vi "commander11.vi"() -> ()   [LabVIEW 2015]
uses:
  <vilib>/National Instruments/NI Dynamixel API/Dynamixel Pro Driver/Controls/Write Select Pro.ctl
  <vilib>/National Instruments/NI Dynamixel API/Dynamixel Pro Driver/Controls/Baudrate Selector.ctl
  G_LCM.vi
  G_ALL.vi
  G_SEN.vi
  <vilib>/National Instruments/NI Dynamixel API/Dynamixel Pro Driver/Write/Write Dynamixel Pro.vi
  <vilib>/National Instruments/NI Dynamixel API/Dynamixel Pro Driver/Helper VIs/Torque Disable.vi
  <vilib>/National Instruments/NI Dynamixel API/Dynamixel Pro Driver/Helper VIs/Torque Enable.vi
  <vilib>/National Instruments/NI Dynamixel API/Dynamixel Pro Driver/Dynamixel Pro Driver.lvlib
panel:
  in  "an":dbl=0.1 format="%#_13g"
  out "Mobileye":bool=TRUE
  in  "Laser lane":bool
  in  "safe  dist":dbl=0.7 format="%#_13g"
  in  "Path Num":i32=1 min=1 max=5 step=1
  out "CIPV_SPEED":dbl=25.0
  out "CIPV_dist":dbl=25.0
  in  "mission":i32
  out "size(s)":i32=1381
  in  "shift torque gain":i32
  out "robotis":refnum<visa-resource-name>
  in  "y 2":dbl=1.0
  in  "y":dbl=0.5 format="%#_13g"
  in  "dist_error_gain":dbl=0.5 format="%#_13g"
  in  "Global y shift":dbl min=-5.0 max=5.0 step=0.1
  in  "d":dbl=-3.5 format="%#_13g"
  in  "reset path":bool
  out "count":i32=100
  out "signal":picture[](array[picture])=[bytes[7530], bytes[7530], bytes[7530], bytes[7530]]
  out "sign":picture[](array[picture])=[bytes[7530], bytes[7530], bytes[7530], bytes[7530]]
  out "trafic signal ref":picture[](array[picture])=[bytes[7530], bytes[7530], bytes[7530], bytes[7530], bytes[7530], bytes[7530]]
  out "sign ref":picture[](array[picture])=[bytes[7530], bytes[7530], bytes[7530], bytes[7530], bytes[7530], bytes[7530], bytes[7530], bytes[7530], bytes[7530], bytes[7530], bytes[7530], bytes[7530], bytes[7530]]
  in  "TTL":bool=TRUE
  in  "lane keep":bool
  in  "replay":bool
  in  "Global x shift":dbl min=-5.0 max=5.0 step=1.0
  out "display":u32=33 format="%02.0f"
  out "control":u32=10 format="%02.0f"
  in  "Vision Lane":bool=TRUE
  in  "save lcm":bool
  out "LCM Recv Data":string
  out "GPS DATA 2":T1={"type"="None", "x_lcc"=0.0, "y_lcc"=0.0, "latdev"=0.0, "londev"=0.0, "sats"=0, "gps_l1_ranges"=0, "gps_l1_mask_ranges"=0, "gps_l2_mask_ranges"=0, "Heading"=0.0, "lon"=0.0, "lat"=0.0, "time"="09:00:00.0", "hgps"=0.0, "lag"=0.0, "MAP"=""} {"lag" format="%#_5g"; "hgps" format="%#_5g"; "lat" format="%#_11g"; "lon" format="%#_11g"; "Heading" format="%#_5g"; "latdev" format="%#_4g"; "londev" format="%#_4g"}
  in  "Obs":bool=TRUE
  in  "Log":bool
  out "path":u32=10 format="%02.0f"
  out "sensor":u32=27 format="%02.0f"
  out "Speed limit":dbl=10.0
  out "collision":bool
  in  "Load Path":bool
  in  "Max. Vel.":dbl=10.0 min=-5.0 max=120.0 step=5.0
  out "col":i16(graph)
  out "stop":bool
  in  "Reverse":bool
  in  "STOP":bool
  out "Waveform Chart 4":cluster{"auto":i16, "run":i16}(graph)={"auto"=1, "run"=0}
  out "Waveform Chart 3":cluster{"Steer_input":dbl, dbl, "handle":dbl}(graph)={"Steer_input"=0.0, -0.0, "handle"=nan}
  out "Waveform Chart 2":T2(graph)={"VS_des"=0.0, "VS_can"=0.0, "VS_des"=10.0}
  out "Heading":cluster{"Heading":dbl, "hgps":dbl}(graph)
  out "XY Graph 2":cluster{"Y":dbl[], "Y":dbl[]}[](graph)
  out "Gauge":cluster{dbl, dbl, dbl}(knob)={0.0, 0.0, 10.0} scale=-20.0..140.0
  out "Meter":cluster{dbl, dbl, dbl}(knob)={0.0, -0.0, nan} scale=-550.0..550.0
  out "XY Graph":cluster{"Y":dbl[], "Y":dbl[]}[](graph)=[{"Y"=[], "Y"=[]}, {"Y"=[-0.0, -0.0, -0.0, -0.0, -0.0, -0.0, -0.0, -0.0, -0.0, -0.0, -0.0, -0.0, -0.0, -0.0, -0.0, -0.0, -0.0, -0.0, -0.0, -0.0, -0.0, -0.0, -0.0, -0.0, -0.0, -0.0, -0.0, -0.0, -0.0, -0.0, -0.0], "Y"=[-4.0, -3.9, -3.8, -3.7, -3.6, -3.5, -3.4, -3.3, -3.2, -3.1, -3.0, -2.9, -2.8, -2.7, -2.5999999999999996, -2.5, -2.4, -2.3, -2.2, -2.0999999999999996, -2.0, -1.9, -1.7999999999999998, -1.6999999999999997, -1.5999999999999996, -1.5, -1.4, -1.2999999999999998, -1.1999999999999997, -1.0999999999999996, -1.0]}, {"Y"=[0.0], "Y"=[0.0]}, {"Y"=[], "Y"=[]}, {"Y"=[-0.925, -0.925, -0.925, -0.6775, -0.6775, -0.925, -0.925, -0.925, -0.925, -0.6775, -0.6775, -0.925, -0.925, -0.925, 0.9025, 0.9025, 0.9025, 0.6775, 0.6775, 0.9025, 0.9025, 0.9025, 0.9025, 0.6775, 0.6775, 0.9025, 0.9025, 0.9025, -0.925], "Y"=[-0.75, -0.224, 0.224, 0.224, -0.224, -0.224, 0.224, 2.415, 2.885, 2.885, 2.415, 2.415, 2.885, 3.5, 3.5, 2.885, 2.415, 2.415, 2.885, 2.885, 2.415, 0.224, -0.224, -0.224, 0.224, 0.224, -0.224, -0.75, -0.75]}, {"Y"=[-0.11693930899008871, -0.11530935243371389, -0.11366872898963808, -0.11201743865786128, -0.11035548143838347, -0.10868285733120467, -0.10699956633632488, -0.10530560845374409, -0.1036009836834623, -0.10188569202547951, -0.10015973347979573, -0.09842310804641094, -0.09667581572532517, -0.09491785651653842, -0.09314923042005063, -0.09136993743586189, -0.08957997756397212, -0.08777935080438137, -0.08596805715708963, -0.08414609662209688, -0.08231346919940313, -0.0804701748890084, -0.07861621369091265, -0.07675158560511593, -0.07487629063161819, -0.07299032877041947, -0.07109370002151975, -0.06918640438491905, -0.06726844186061733, -0.06533981244861461, -0.06340051614891093, -0.061450552961506213, -0.05948992288640052, -0.05751862592359382, -0.055536662073086135, -0.05354403133487746, -0.05154073370896778, -0.0495267691953571, -0.04750213779404542, -0.045466839505032754, -0.04342087432831909, -0.04136424226390442, -0.03929694331178877, -0.03721897747197212, -0.035130344744454464, -0.033031045129235825, -0.03092107862631617, -0.028800445235695537, -0.02666914495737389, -0.024527177791351266, -0.02237454373762765, -0.02021124279620301, -0.018037274967077403, -0.015852640250250776, -0.013657338645723171, -0.011451370153494574, -0.009234734773564957, -0.007007432505934365, -0.004769463350602757, -0.002520827307570167, -0.0002615243768365888, 0.0020084454415980058, 0.004289082147733582, 0.0065803857415701675, 0.008882356223107735, 0.011194993592346297, 0.013518297849285876, 0.01585226899392643, 0.018196907026268, 0.020552211946310545, 0.02291818375405409, 0.025294822449498655, 0.02768212803264418, 0.03008010050349072, 0.03248873986203825, 0.03490804610828678, 0.037338019242236314, 0.03977865926388684, 0.04222996617323836, 0.044691939970290875, 0.04716458065504438, 0.04964788822749888, 0.05214186268765442, 0.05464650403551091, 0.057161812271068396, 0.05968778739432688, 0.06222442940528636, 0.06477173830394688, 0.06732971409030836, 0.06989835676437083, 0.07247766632613428, 0.07506764277559874, 0.07766828611276426, 0.08027959633763071, 0.08290157345019813, 0.08553421745046658, 0.08817752833843606, 0.09083150611410651, 0.09349615077747794, 0.09617146232855037, 0.0988574407673238], "Y"=[-4.0, -3.9, -3.8, -3.7, -3.6, -3.5, -3.4, -3.3, -3.2, -3.1, -3.0, -2.9, -2.8, -2.7, -2.5999999999999996, -2.5, -2.4, -2.3, -2.2, -2.0999999999999996, -2.0, -1.9, -1.7999999999999998, -1.6999999999999997, -1.5999999999999996, -1.5, -1.4, -1.2999999999999998, -1.1999999999999997, -1.0999999999999996, -1.0, -0.8999999999999999, -0.7999999999999998, -0.6999999999999997, -0.5999999999999996, -0.5, -0.3999999999999999, -0.2999999999999998, -0.19999999999999973, -0.09999999999999964, 0.0, 0.10000000000000053, 0.20000000000000018, 0.2999999999999998, 0.40000000000000036, 0.5, 0.6000000000000005, 0.7000000000000002, 0.8000000000000007, 0.9000000000000004, 1.0, 1.1000000000000005, 1.2000000000000002, 1.3000000000000007, 1.4000000000000004, 1.5, 1.6000000000000005, 1.7000000000000002, 1.8000000000000007, 1.9000000000000004, 2.0, 2.1000000000000005, 2.2, 2.3000000000000007, 2.4000000000000004, 2.5, 2.6000000000000005, 2.7, 2.8000000000000007, 2.9000000000000004, 3.0, 3.1000000000000005, 3.2, 3.3000000000000007, 3.4000000000000004, 3.5, 3.6000000000000005, 3.7, 3.8000000000000007, 3.9000000000000004, 4.0, 4.1, 4.200000000000001, 4.300000000000001, 4.4, 4.5, 4.6, 4.700000000000001, 4.800000000000001, 4.9, 5.0, 5.1, 5.200000000000001, 5.300000000000001, 5.4, 5.5, 5.600000000000001, 5.700000000000001, 5.800000000000001, 5.9, 6.0]}, {"Y"=[0.8254985256386238, 0.8528194590155173, 0.8796538166129886, 0.9060015984310377, 0.9318628044696647, 0.9572374347288698, 0.9821254892086528, 1.0065269679090136, 1.0304418708299523, 1.0538701979714689, 1.0768119493335635, 1.099267124916236, 1.1212357247194864, 1.1427177487433147, 1.163713196987721, 1.184222069452705, 1.204244366138267, 1.2237800870444069, 1.2428292321711245, 1.2613918015184205, 1.279467795086294, 1.2970572128747455, 1.314160054883775, 1.3307763211133825, 1.3469060115635676, 1.3625491262343308, 1.3777056651256718, 1.392375628237591, 1.4065590155700878, 1.4202558271231627, 1.4334660628968152, 1.4461897228910459, 1.4584268071058544, 1.4701773155412408, 1.4814412481972052, 1.4922186050737474, 1.5025093861708676, 1.5123135914885657, 1.5216312210268417, 1.5304622747856955, 1.5388067527651272, 1.546664654965137, 1.5540359813857245, 1.56092073202689, 1.5673189068886335, 1.5732305059709548, 1.578655529273854, 1.583593976797331, 1.5880458485413862, 1.592011144506019, 1.5954898646912299, 1.5984820090970187, 1.6009875777233853, 1.60300657057033, 1.6045389876378524, 1.605584828925953, 1.606144094434631, 1.6062167841638872, 1.6058028981137213, 1.6049024362841335, 1.6035153986751234, 1.601641785286691, 1.599281596118837, 1.5964348311715606, 1.5931014904448622, 1.5892815739387416, 1.584975081653199, 1.5801820135882343, 1.5749023697438473, 1.5691361501200385, 1.5628833547168075, 1.5561439835341544, 1.5489180365720792, 1.541205513830582, 1.5330064153096625, 1.5243207410093211, 1.5151484909295576, 1.505489665070372, 1.4953442634317642, 1.4847122860137343, 1.4735937328162825, 1.4619886038394085, 1.4498968990831123, 1.437318618547394, 1.4242537622322538, 1.4107023301376915, 1.396664322263707, 1.3821397386103003, 1.3671285791774717, 1.351630843965221, 1.335646532973548, 1.3191756462024533, 1.302218183651936, 1.284774145321997, 1.2668435312126356, 1.2484263413238526, 1.229522575655647, 1.2101322342080194, 1.19025531698097, 1.1698918239744982, 1.1490417551886045], "Y"=[-4.0, -3.9, -3.8, -3.7, -3.6, -3.5, -3.4, -3.3, -3.2, -3.1, -3.0, -2.9, -2.8, -2.7, -2.5999999999999996, -2.5, -2.4, -2.3, -2.2, -2.0999999999999996, -2.0, -1.9, -1.7999999999999998, -1.6999999999999997, -1.5999999999999996, -1.5, -1.4, -1.2999999999999998, -1.1999999999999997, -1.0999999999999996, -1.0, -0.8999999999999999, -0.7999999999999998, -0.6999999999999997, -0.5999999999999996, -0.5, -0.3999999999999999, -0.2999999999999998, -0.19999999999999973, -0.09999999999999964, 0.0, 0.10000000000000053, 0.20000000000000018, 0.2999999999999998, 0.40000000000000036, 0.5, 0.6000000000000005, 0.7000000000000002, 0.8000000000000007, 0.9000000000000004, 1.0, 1.1000000000000005, 1.2000000000000002, 1.3000000000000007, 1.4000000000000004, 1.5, 1.6000000000000005, 1.7000000000000002, 1.8000000000000007, 1.9000000000000004, 2.0, 2.1000000000000005, 2.2, 2.3000000000000007, 2.4000000000000004, 2.5, 2.6000000000000005, 2.7, 2.8000000000000007, 2.9000000000000004, 3.0, 3.1000000000000005, 3.2, 3.3000000000000007, 3.4000000000000004, 3.5, 3.6000000000000005, 3.7, 3.8000000000000007, 3.9000000000000004, 4.0, 4.1, 4.200000000000001, 4.300000000000001, 4.4, 4.5, 4.6, 4.700000000000001, 4.800000000000001, 4.9, 5.0, 5.1, 5.200000000000001, 5.300000000000001, 5.4, 5.5, 5.600000000000001, 5.700000000000001, 5.800000000000001, 5.9, 6.0]}, {"Y"=[-1.0593771436188013, -1.0834381638829451, -1.1069912745922648, -1.1300364757467602, -1.1525737673464316, -1.1746031493912792, -1.1961246218813026, -1.2171381848165017, -1.2376438381968768, -1.257641582022428, -1.277131416293155, -1.296113341009058, -1.314587356170137, -1.3325534617763914, -1.3500116578278223, -1.3669619443244287, -1.3834043212662113, -1.3993387886531696, -1.4147653464853038, -1.4296839947626143, -1.4440947334851004, -1.4579975626527624, -1.4713924822656004, -1.4842794923236142, -1.4966585928268041, -1.5085297837751699, -1.5198930651687115, -1.530748437007429, -1.5410958992913224, -1.5509354520203917, -1.5602670951946371, -1.5690908288140584, -1.5774066528786554, -1.5852145673884286, -1.5925145723433776, -1.5993066677435024, -1.605590853588803, -1.6113671298792798, -1.6166354966149326, -1.621395953795761, -1.6256485014217654, -1.6293931394929457, -1.632629868009302, -1.6353586869708343, -1.6375795963775424, -1.6392925962294265, -1.6404976865264864, -1.6411948672687222, -1.6413841384561338, -1.6410655000887215, -1.6402389521664853, -1.6389044946894247, -1.6370621276575401, -1.6347118510708316, -1.6318536649292987, -1.628487569232942, -1.624613563981761, -1.620231649175756, -1.615341824814927, -1.6099440908992737, -1.6040384474287965, -1.5976248944034952, -1.5907034318233697, -1.5832740596884203, -1.5753367779986467, -1.566891586754049, -1.5579384859546273, -1.5484774756003814, -1.5385085556913114, -1.5280317262274175, -1.5170469872086993, -1.505554338635157, -1.4935537805067909, -1.4810453128236005, -1.4680289355855862, -1.4545046487927475, -1.440472452445085, -1.4259323465425984, -1.4108843310852874, -1.3953284060731526, -1.3792645715061937, -1.3626928273844108, -1.3456131737078034, -1.3280256104763721, -1.309930137690117, -1.2913267553490377, -1.2722154634531344, -1.2525962620024065, -1.232469150996855, -1.2118341304364795, -1.1906912003212795, -1.1690403606512558, -1.1468816114264073, -1.1242149526467355, -1.1010403843122396, -1.077357906422919, -1.0531675189787748, -1.0284692219798064, -1.0032630154260138, -0.9775488993173974, -0.9513268736539569], "Y"=[-4.0, -3.9, -3.8, -3.7, -3.6, -3.5, -3.4, -3.3, -3.2, -3.1, -3.0, -2.9, -2.8, -2.7, -2.5999999999999996, -2.5, -2.4, -2.3, -2.2, -2.0999999999999996, -2.0, -1.9, -1.7999999999999998, -1.6999999999999997, -1.5999999999999996, -1.5, -1.4, -1.2999999999999998, -1.1999999999999997, -1.0999999999999996, -1.0, -0.8999999999999999, -0.7999999999999998, -0.6999999999999997, -0.5999999999999996, -0.5, -0.3999999999999999, -0.2999999999999998, -0.19999999999999973, -0.09999999999999964, 0.0, 0.10000000000000053, 0.20000000000000018, 0.2999999999999998, 0.40000000000000036, 0.5, 0.6000000000000005, 0.7000000000000002, 0.8000000000000007, 0.9000000000000004, 1.0, 1.1000000000000005, 1.2000000000000002, 1.3000000000000007, 1.4000000000000004, 1.5, 1.6000000000000005, 1.7000000000000002, 1.8000000000000007, 1.9000000000000004, 2.0, 2.1000000000000005, 2.2, 2.3000000000000007, 2.4000000000000004, 2.5, 2.6000000000000005, 2.7, 2.8000000000000007, 2.9000000000000004, 3.0, 3.1000000000000005, 3.2, 3.3000000000000007, 3.4000000000000004, 3.5, 3.6000000000000005, 3.7, 3.8000000000000007, 3.9000000000000004, 4.0, 4.1, 4.200000000000001, 4.300000000000001, 4.4, 4.5, 4.6, 4.700000000000001, 4.800000000000001, 4.9, 5.0, 5.1, 5.200000000000001, 5.300000000000001, 5.4, 5.5, 5.600000000000001, 5.700000000000001, 5.800000000000001, 5.9, 6.0]}, {"Y"=[], "Y"=[]}, {"Y"=[0.0], "Y"=[0.0]}, {"Y"=[], "Y"=[]}, {"Y"=[], "Y"=[]}, {"Y"=[0.0], "Y"=[0.0]}, {"Y"=[-2.34, -2.34, -2.34, -2.34, -2.2800000000000002, -2.2800000000000002, -2.2800000000000002, -2.2800000000000002, -2.22, -2.22, -2.22, -2.16, -2.16, -2.16, -2.1, -2.1, -2.1, -2.04, -2.04, -2.04, -2.04, -1.98, -1.98, -1.98, -1.98, -1.68, -1.68, -1.68, -1.68, -1.68, -1.68, -1.68, -1.68, -1.68, -1.68, -1.68, -1.68, -1.68, -1.68, -1.68, -1.68, -1.68, -1.68, -1.68, -1.68, -1.68, -1.68, -1.68, -1.68, -1.68, -1.68, -1.68, -1.68, -1.68, -1.68, -1.68, -1.68, -1.68, -1.68, -1.68, -1.68, -1.68, -1.68, -1.68, -1.68, -1.68, -1.68, -1.62, -1.62, -1.62, -1.62, -1.62, -1.62, -1.62, -1.62, -1.62, -1.62, -1.62, -1.62, -1.62, -1.62, -1.62, -1.62, -1.62, -1.62, -1.62, -1.62, -1.62, -1.62, -1.62, -1.62, -1.62, -1.62, -1.62, -1.62, -1.62, -1.62, -1.62, -1.62, -1.62, -1.62, -1.62, -1.62, -1.62, -1.62, -1.62, -1.62, -1.62, -1.62, -1.62, -1.62, -1.62, -1.62, -1.62, -1.62, -1.62, -1.62, -1.62, -1.62, -1.62, -1.62, -1.62, -1.62, -1.62, -1.62, -1.62, -1.62, -1.62, -1.62, -1.62, -1.62, -1.62, -1.62, -1.62, -1.62, -1.62, -1.62, -1.62, -1.62, -1.62, -1.62, -1.62, -1.62, -1.62, -1.62, -1.62, -1.62, -1.56, -1.56, -1.56, -1.56, -1.56, -1.56, -1.56, -1.56, -1.56, -1.56, -1.56, -1.56, -1.56, -1.56, -1.56, -1.56, -1.56, -1.56, -1.56, -1.56, -1.56, -1.56, -1.56, -1.56, -1.56, -1.56, -1.56, -1.56, -1.56, -1.56, -1.56, -1.56, -1.56, -1.56, -1.56, -1.56, -1.56, -1.56, -1.56, -1.56, -1.56, -1.56, -1.56, -1.56, -1.56, -1.56, -1.56, -1.56, -1.56, -1.56, -1.56, -1.56, -1.56, -1.56, -1.56, -1.56, -1.56, -1.56, -1.56, -1.56, -1.56, -1.56, -1.56, -1.56, -1.56, -1.56, -1.56, -1.56, -1.56, -1.56, -1.56, -1.56, -1.56, -1.56, -1.56, -1.56, -1.56, -1.56, -1.56, -1.56, -1.56, -1.56, -1.56, -1.56, -1.56, -1.56, -1.56, -1.56, -1.56, -1.56, -1.56, -1.56, -1.56, -1.56, -1.5, -1.5, -1.5, -1.5, -1.5, -1.5, -1.5, -1.5, -1.5, -1.5, -1.5, -1.5, -1.5, -1.5, -1.5, -1.5, -1.5, -1.5, -1.5, -1.5, -1.5, -1.5, -1.5, -1.5, -1.5, -1.5, -1.5, -1.5, -1.5, -1.5, -1.5, -1.5, -1.5, -1.5, -1.5, -1.5, -1.5, -1.5, -1.5, -1.5, -1.5, -1.5, -1.5, -1.5, -1.5, -1.5, -1.5, -1.5, -1.5, -1.5, -1.44, -1.44, -1.44, -1.44, -1.44, -1.44, -1.44, -1.44, -1.44, -1.44, -1.44, -1.44, -1.44, -1.44, -1.44, -1.44, -1.44, -1.44, -1.44, -1.44, -1.44, -1.44, -1.44, -1.44, -1.44, -1.44, -1.44, -1.44, -1.44, -1.44, -1.44, -1.44, -1.44, -1.44, -1.3800000000000001, -1.3800000000000001, -1.3800000000000001, -1.3800000000000001, -1.3800000000000001, -1.3800000000000001, -1.3800000000000001, -1.3800000000000001, -1.3800000000000001, -1.3800000000000001, -1.3800000000000001, -1.3800000000000001, -1.3800000000000001, -1.3800000000000001, -1.3800000000000001, -1.3800000000000001, -1.3800000000000001, -1.3800000000000001, -1.3800000000000001, -1.3800000000000001, -1.3800000000000001, -1.32, -1.32, -1.32, -1.32, -1.32, -1.32, -1.32, -1.32, -1.32, -1.32, -1.32, -1.32, -1.32, -1.32, -1.32, -1.32, -1.32, -1.32, -1.32, -1.32, -1.32, -1.26, -1.26, -1.26, -1.26, -1.26, -1.26, -1.26, -1.26, -1.26, -1.26, -1.26, -1.26, -1.26, -1.26, -1.26, -1.26, -1.26, -1.26, -1.26, -1.26, -1.26, -1.26, -1.26, -1.26, -1.26, -1.26, -1.26, -1.26, -1.2, -1.2, -1.2, -1.2, -1.2, -1.2, -1.2, -1.2, -1.2, -1.2, -1.2, -1.2, -1.2, -1.2, -1.2, -1.2, -1.2, -1.2, -1.2, -1.2, -1.2, -1.2, -1.2, -1.2, -1.2, -1.2, -1.2, -1.2, -1.2, -1.1400000000000001, -1.1400000000000001, -1.1400000000000001, -1.1400000000000001, -1.1400000000000001, -1.1400000000000001, -1.1400000000000001, -1.1400000000000001, -1.1400000000000001, -1.1400000000000001, -1.1400000000000001, -1.1400000000000001, -1.1400000000000001, -1.1400000000000001, -1.1400000000000001, -1.1400000000000001, -1.1400000000000001, -1.1400000000000001, -1.1400000000000001, -1.1400000000000001, -1.1400000000000001, -1.1400000000000001, -1.1400000000000001, -1.1400000000000001, -1.1400000000000001, -1.1400000000000001, -1.1400000000000001, -1.08, -1.08, -1.08, -1.08, -1.08, -1.08, -1.08, -1.08, -1.08, -1.08, -1.08, -1.08, -1.08, -1.08, -1.08, -1.08, -1.08, -1.08, -1.08, -1.08, -1.08, -1.02, -1.02, -1.02, -1.02, -1.02, -1.02, -1.02, -1.02, -1.02, -1.02, -1.02, -1.02, -1.02, -1.02, -1.02, -1.02, -1.02, -1.02, -1.02, -1.02, -0.96, -0.96, -0.96, -0.96, -0.96, -0.96, -0.96, -0.96, -0.96, -0.96, -0.96, -0.96, -0.96, -0.96, -0.96, -0.96, -0.96, -0.96, -0.96, -0.96, -0.96, -0.96, -0.96, -0.96, -0.96, -0.96, -0.9, -0.9, -0.9, -0.9, -0.9, -0.9, -0.9, -0.9, -0.9, -0.9, -0.9, -0.9, -0.9, -0.9, -0.9, -0.9, -0.9, -0.9, -0.9, -0.9, -0.9, -0.9, -0.9, -0.9, -0.9, -0.9, -0.9, -0.84, -0.84, -0.84, -0.84, -0.84, -0.84, -0.84, -0.84, -0.84, -0.84, -0.84, -0.84, -0.84, -0.84, -0.84, -0.84, -0.84, -0.84, -0.84, -0.84, -0.84, -0.84, -0.84, -0.84, -0.84, -0.84, -0.84, -0.78, -0.78, -0.78, -0.78, -0.78, -0.78, -0.78, -0.78, -0.78, -0.78, -0.78, -0.78, -0.78, -0.78, -0.78, -0.78, -0.78, -0.78, -0.78, -0.78, -0.78, -0.78, -0.78, -0.78, -0.72, -0.72, -0.72, -0.72, -0.72, -0.72, -0.72, -0.72, -0.72, -0.72, -0.72, -0.72, -0.72, -0.72, -0.72, -0.72, -0.72, -0.72, -0.72, -0.72, -0.72, -0.72, -0.66, -0.66, -0.66, -0.66, -0.66, -0.66, -0.66, -0.66, -0.66, -0.66, -0.66, -0.66, -0.66, -0.66, -0.66, -0.66, -0.66, -0.66, -0.66, -0.66, -0.66, -0.66, -0.66, -0.66, -0.66, -0.66, -0.66, -0.66, -0.66, -0.66, -0.66, -0.66, -0.66, -0.66, -0.6, -0.6, -0.6, -0.6, -0.6, -0.6, -0.6, -0.6, -0.6, -0.6, -0.6, -0.6, -0.6, -0.6, -0.6, -0.6, -0.6, -0.6, -0.6, -0.6, -0.6, -0.6, -0.6, -0.6, -0.6, -0.6, -0.6, -0.54, -0.54, -0.54, -0.54, -0.54, -0.54, -0.54, -0.54, -0.54, -0.54, -0.54, -0.54, 0.54, 0.54, 0.54, 0.54, 0.54, 0.54, 0.54, 0.54, 0.54, 0.6, 0.6, 0.6, 0.6, 0.6, 0.6, 0.6, 0.6, 0.6, 0.6, 0.6, 0.6, 0.6, 0.66, 0.66, 0.66, 0.66, 0.66, 0.66, 0.66, 0.66, 0.66, 0.66, 0.66, 0.66, 0.66, 0.66, 0.72, 0.72, 0.72, 0.72, 0.72, 0.72, 0.72, 0.72, 0.72, 0.78, 0.78, 0.78, 0.78, 0.78, 0.78, 0.78, 0.78, 0.78, 0.78, 0.78, 0.78, 0.84, 0.84, 0.84, 0.84, 0.84, 0.84, 0.84, 0.84, 0.84, 0.84, 0.84, 0.84, 0.9, 0.9, 0.9, 0.9, 0.9, 0.9, 0.9, 0.9, 0.9, 0.9, 0.9, 0.9, 0.9, 0.9, 0.9, 0.9, 0.9, 0.9, 0.9, 0.9, 0.96, 0.96, 0.96, 0.96, 0.96, 0.96, 0.96, 0.96, 0.96, 0.96, 0.96, 0.96, 0.96, 0.96, 0.96, 0.96, 0.96, 0.96, 0.96, 0.96, 0.96, 0.96, 0.96, 0.96, 0.96, 0.96, 0.96, 0.96, 1.02, 1.02, 1.02, 1.02, 1.02, 1.02, 1.02, 1.02, 1.02, 1.02, 1.02, 1.02, 1.02, 1.02, 1.02, 1.02, 1.02, 1.02, 1.02, 1.02, 1.02, 1.02, 1.02, 1.02, 1.02, 1.02, 1.02, 1.02, 1.02, 1.02, 1.02, 1.02, 1.08, 1.08, 1.08, 1.08, 1.08, 1.08, 1.08, 1.08, 1.08, 1.08, 1.08, 1.08, 1.08, 1.08, 1.08, 1.08, 1.08, 1.08, 1.08, 1.08, 1.08, 1.08, 1.08, 1.08, 1.08, 1.08, 1.08, 1.08, 1.08, 1.08, 1.08, 1.08, 1.08, 1.08, 1.08, 1.08, 1.1400000000000001, 1.1400000000000001, 1.1400000000000001, 1.1400000000000001, 1.1400000000000001, 1.1400000000000001, 1.1400000000000001, 1.1400000000000001, 1.1400000000000001, 1.1400000000000001, 1.1400000000000001, 1.1400000000000001, 1.1400000000000001, 1.1400000000000001, 1.1400000000000001, 1.1400000000000001, 1.1400000000000001, 1.1400000000000001, 1.1400000000000001, 1.1400000000000001, 1.1400000000000001, 1.1400000000000001, 1.1400000000000001, 1.1400000000000001, 1.1400000000000001, 1.1400000000000001, 1.1400000000000001, 1.1400000000000001, 1.1400000000000001, 1.1400000000000001, 1.1400000000000001, 1.1400000000000001, 1.1400000000000001, 1.1400000000000001, 1.1400000000000001, 1.1400000000000001, 1.1400000000000001, 1.2, 1.2, 1.2, 1.2, 1.2, 1.2, 1.2, 1.2, 1.2, 1.2, 1.2, 1.2, 1.2, 1.2, 1.2, 1.2, 1.2, 1.2, 1.2, 1.2, 1.2, 1.2, 1.2, 1.2, 1.2, 1.2, 1.2, 1.2, 1.2, 1.26, 1.26, 1.26, 1.26, 1.26, 1.26, 1.26, 1.26, 1.26, 1.26, 1.26, 1.26, 1.26, 1.26, 1.26, 1.26, 1.26, 1.26, 1.26, 1.26, 1.26, 1.26, 1.26, 1.26, 1.26, 1.26, 1.26, 1.26, 1.26, 1.26, 1.26, 1.26, 1.26, 1.26, 1.32, 1.32, 1.32, 1.32, 1.32, 1.32, 1.32, 1.32, 1.32, 1.32, 1.32, 1.32, 1.32, 1.32, 1.32, 1.32, 1.32, 1.32, 1.32, 1.32, 1.32, 1.32, 1.32, 1.32, 1.32, 1.32, 1.32, 1.32, 1.32, 1.32, 1.32, 1.32, 1.32, 1.32, 1.32, 1.3800000000000001, 1.3800000000000001, 1.3800000000000001, 1.3800000000000001, 1.3800000000000001, 1.3800000000000001, 1.3800000000000001, 1.3800000000000001, 1.3800000000000001, 1.3800000000000001, 1.3800000000000001, 1.3800000000000001, 1.3800000000000001, 1.3800000000000001, 1.3800000000000001, 1.3800000000000001, 1.3800000000000001, 1.3800000000000001, 1.3800000000000001, 1.3800000000000001, 1.3800000000000001, 1.3800000000000001, 1.3800000000000001, 1.3800000000000001, 1.3800000000000001, 1.3800000000000001, 1.3800000000000001, 1.3800000000000001, 1.3800000000000001, 1.3800000000000001, 1.3800000000000001, 1.3800000000000001, 1.3800000000000001, 1.3800000000000001, 1.3800000000000001, 1.44, 1.44, 1.44, 1.44, 1.44, 1.44, 1.44, 1.44, 1.44, 1.44, 1.44, 1.44, 1.44, 1.44, 1.44, 1.44, 1.44, 1.44, 1.44, 1.44, 1.44, 1.44, 1.44, 1.44, 1.44, 1.44, 1.44, 1.44, 1.44, 1.44, 1.44, 1.44, 1.44, 1.44, 1.44, 1.44, 1.44, 1.44, 1.44, 1.44, 1.5, 1.5, 1.5, 1.5, 1.5, 1.5, 1.5, 1.5, 1.5, 1.5, 1.5, 1.5, 1.5, 1.5, 1.5, 1.5, 1.5, 1.5, 1.5, 1.5, 1.5, 1.5, 1.5, 1.5, 1.5, 1.5, 1.5, 1.5, 1.5, 1.5, 1.5, 1.5, 1.5, 1.5, 1.5, 1.5, 1.5, 1.5, 1.5, 1.5, 1.5, 1.5, 1.5, 1.5, 1.5, 1.5, 1.5, 1.5, 1.5, 1.5, 1.5, 1.5, 1.5, 1.5, 1.5, 1.5, 1.5, 1.5, 1.5, 1.5, 1.5, 1.5, 1.5, 1.56, 1.56, 1.56, 1.56, 1.56, 1.56, 1.56, 1.56, 1.56, 1.56, 1.56, 1.56, 1.56, 1.56, 1.56, 1.56, 1.56, 1.56, 1.56, 1.56, 1.56, 1.56, 1.56, 1.56, 1.56, 1.56, 1.56, 1.56, 1.56, 1.56, 1.56, 1.56, 1.56, 1.56, 1.56, 1.56, 1.56, 1.56, 1.56, 1.56, 1.56, 1.56, 1.56, 1.56, 1.56, 1.56, 1.56, 1.56, 1.56, 1.56, 1.56, 1.56, 1.56, 1.56, 1.56, 1.56, 1.56, 1.56, 1.56, 1.56, 1.56, 1.56, 1.56, 1.56, 1.56, 1.56, 1.56, 1.56, 1.56, 1.56, 1.56, 1.56, 1.56, 1.56, 1.56, 1.56, 1.56, 1.56, 1.56, 1.56, 1.56, 1.56, 1.56, 1.56, 1.56, 1.62, 1.62, 1.62, 1.62, 1.62, 1.62, 1.62, 1.62, 1.62, 1.62, 1.62, 1.62, 1.62, 1.62, 1.62, 1.62, 1.62, 1.62, 1.62, 1.62, 1.62, 1.62, 1.62, 1.62, 1.62, 1.62, 1.62, 1.62, 1.62, 1.62, 1.62, 1.62, 1.62, 1.62, 1.62, 1.62, 1.62, 1.62, 1.62, 1.62, 1.62, 1.62, 1.62, 1.62, 1.62, 1.62, 1.62, 1.62, 1.62, 1.62, 1.62, 1.62, 1.62, 1.62, 1.62, 1.62, 1.62, 1.62, 1.62, 1.62, 1.62, 1.62, 1.62, 1.62, 1.62, 1.62, 1.62, 1.62, 1.62, 1.62, 1.62, 1.62, 1.68, 1.68, 1.68, 1.68, 1.68, 1.68, 1.68, 1.68, 1.68, 1.68, 1.68, 1.68, 1.68, 1.68, 1.74, 1.74, 1.74, 1.74, 1.74, 1.8, 1.8, 1.8, 1.8, 1.8, 1.8, 1.86, 1.86, 1.86, 1.86, 1.92, 1.92, 1.92, 1.92, 1.92, 1.98, 1.98, 1.98, 1.98, 1.98, 1.98, 2.04, 2.04, 2.04, 2.04, 2.04, 2.1, 2.1, 2.1, 2.1, 2.1, 2.16, 2.16, 2.16, 2.16, 2.22, 2.22, 2.22, 2.22, 2.2800000000000002, 2.2800000000000002, 2.2800000000000002, 2.2800000000000002, 2.2800000000000002, 2.2800000000000002, 2.2800000000000002, 2.34, 2.34, 2.34, 2.34, 2.34, 2.34, 2.34, 2.34, 2.34, 2.34], "Y"=[-5.88, -5.94, -6.0, -6.0600000000000005, -5.88, -5.94, -6.0, -6.0600000000000005, -5.88, -5.94, -6.0, -6.3, -6.36, -6.42, -6.3, -6.36, -6.42, -6.24, -6.3, -6.36, -6.42, -6.24, -6.3, -6.36, -6.42, 2.04, 1.98, 1.92, 1.86, 1.8, 1.74, 1.68, 1.62, 1.56, 1.5, 1.3800000000000001, 1.32, 1.26, 1.2, 1.1400000000000001, 1.08, 1.02, 0.96, 0.9, 0.84, 0.78, 0.72, 0.66, 0.6, 0.54, 0.48, 0.42, 0.36, 0.3, 0.24, 0.18, 0.12, 0.06, -0.0, -0.06, -0.12, -0.18, -0.24, -0.3, -0.36, -0.42, -0.48, 3.24, 3.18, 3.12, 3.06, 3.0, 2.94, 2.88, 2.82, 2.7600000000000002, 2.7, 2.64, 2.58, 2.52, 2.46, 2.4, 2.34, 2.2800000000000002, 2.22, 2.16, 2.1, 2.04, 1.98, 1.92, 1.86, 1.8, 1.74, 1.68, 1.62, 1.56, 1.5, 1.44, 1.3800000000000001, 1.32, 1.26, 1.2, 1.1400000000000001, 1.08, 1.02, 0.96, 0.9, 0.84, 0.78, 0.72, 0.66, 0.6, 0.54, 0.48, 0.42, 0.36, 0.3, 0.24, 0.18, 0.12, 0.06, -0.0, -0.06, -0.12, -0.18, -0.24, -0.3, -0.36, -0.42, -0.48, -0.54, -0.6, -0.66, -0.72, -0.78, -0.84, -0.9, -0.96, -1.02, -1.08, -1.1400000000000001, -1.2, -1.26, -1.32, -1.3800000000000001, -1.44, -1.5, 3.72, 3.66, 3.6, 3.54, 3.48, 3.42, 3.36, 3.3000000000000003, 3.24, 3.18, 3.12, 3.06, 3.0, 2.94, 2.88, 2.82, 2.7600000000000002, 2.7, 2.64, 2.58, 2.52, 2.46, 2.4, 2.34, 2.2800000000000002, 2.22, 2.16, 2.1, 2.04, 1.98, 1.92, 1.86, 1.8, 1.74, 1.68, 1.62, 1.56, 1.5, 1.44, 1.3800000000000001, 1.32, 1.26, 1.2, 1.1400000000000001, 1.08, 1.02, 0.96, 0.9, 0.84, 0.78, 0.72, 0.66, 0.6, 0.54, 0.48, 0.42, 0.36, 0.3, 0.24, 0.18, 0.12, 0.06, -0.0, -0.06, -0.12, -0.18, -0.24, -0.3, -0.36, -0.42, -0.48, -0.54, -0.6, -0.66, -0.72, -0.78, -0.84, -0.9, -0.96, -1.02, -1.08, -1.1400000000000001, -1.2, -1.26, -1.32, -1.3800000000000001, -1.44, -1.5, -1.56, -1.62, -1.68, -1.74, -1.8, -1.86, 3.72, 3.66, 3.6, 3.54, 3.48, 3.42, 3.36, 3.3000000000000003, 3.24, 3.18, 3.12, 3.06, 3.0, 2.94, 2.88, 2.82, 2.7600000000000002, 2.7, 2.64, 2.58, 2.52, 2.46, 2.4, 2.34, -0.54, -0.6, -0.66, -0.84, -0.9, -0.96, -1.02, -1.08, -1.1400000000000001, -1.2, -1.26, -1.32, -1.3800000000000001, -1.44, -1.5, -1.56, -1.62, -1.68, -1.74, -1.8, -1.86, -1.92, -1.98, -2.04, -2.1, -2.16, 3.96, 3.9, 3.84, 3.7800000000000002, 3.72, 3.66, 3.6, 3.54, 3.48, 3.42, 3.36, 3.3000000000000003, 3.24, 3.18, 3.12, -1.44, -1.5, -1.56, -1.62, -1.68, -1.74, -1.8, -1.86, -1.92, -1.98, -2.04, -2.1, -2.16, -2.22, -2.2800000000000002, -2.34, -2.4, -2.46, -2.52, 4.2, 4.14, 4.08, 4.0200000000000005, 3.96, 3.9, 3.84, 3.7800000000000002, 3.72, 3.66, -1.98, -2.04, -2.1, -2.16, -2.22, -2.2800000000000002, -2.34, -2.4, -2.46, -2.52, -2.58, 4.5600000000000005, 4.5, 4.44, 4.38, 4.32, 4.26, 4.2, 4.14, 4.08, 4.0200000000000005, 3.96, -2.34, -2.4, -2.46, -2.52, -2.58, -2.64, -2.7, -2.7600000000000002, -2.82, -2.88, 4.92, 4.86, 4.8, 4.74, 4.68, 4.62, 4.5600000000000005, 4.5, 4.44, 4.38, 4.32, 4.26, 4.2, -2.52, -2.58, -2.64, -2.7, -2.7600000000000002, -2.82, -2.88, -2.94, -3.0, -3.06, -3.12, -3.18, -3.24, -3.3000000000000003, -3.36, 5.16, 5.1000000000000005, 5.04, 4.98, 4.92, 4.86, 4.8, 4.74, 4.68, 4.62, 4.5600000000000005, 4.5, 4.44, 4.38, -2.94, -3.0, -3.06, -3.12, -3.18, -3.24, -3.3000000000000003, -3.36, -3.42, -3.48, -3.54, -3.6, -3.66, -3.72, -3.7800000000000002, 5.64, 5.58, 5.5200000000000005, 5.46, 5.4, 5.34, 5.28, 5.22, 5.16, 5.1000000000000005, 5.04, 4.98, 4.92, 4.86, 4.8, -3.36, -3.42, -3.48, -3.54, -3.6, -3.66, -3.72, -3.7800000000000002, -3.84, -3.9, -3.96, -4.0200000000000005, 6.0, 5.94, 5.88, 5.82, 5.76, 5.7, 5.64, 5.58, 5.5200000000000005, 5.46, 5.4, 5.34, 5.28, 5.22, -3.84, -3.9, -3.96, -4.0200000000000005, -4.08, -4.14, -4.2, 6.24, 6.18, 6.12, 6.0600000000000005, 6.0, 5.94, 5.88, 5.82, 5.76, 5.7, 5.64, 5.58, 5.5200000000000005, -4.14, -4.2, -4.26, -4.32, -4.38, -4.44, -4.5, 6.72, 6.66, 6.6000000000000005, 6.54, 6.48, 6.42, 6.36, 6.3, 6.24, 6.18, 6.12, 6.0600000000000005, 6.0, 5.94, -4.2, -4.26, -4.32, -4.38, -4.44, -4.5, -4.5600000000000005, -4.62, -4.68, -4.74, -4.8, -4.86, 7.2, 7.140000000000001, 7.08, 7.0200000000000005, 6.96, 6.9, 6.84, 6.78, 6.72, 6.66, 6.6000000000000005, 6.54, 6.48, 6.42, 6.36, 6.3, -4.44, -4.5, -4.5600000000000005, -4.62, -4.68, -4.74, -4.8, -4.86, -4.92, -4.98, -5.04, 7.5600000000000005, 7.5, 7.44, 7.38, 7.32, 7.26, 7.2, 7.140000000000001, 7.08, 7.0200000000000005, 6.96, 6.9, 6.84, 6.78, 6.72, 6.66, 6.6000000000000005, -4.74, -4.8, -4.86, -4.92, -4.98, -5.04, -5.1000000000000005, -5.16, -5.22, -5.28, 7.86, 7.8, 7.74, 7.68, 7.62, 7.5600000000000005, 7.5, 7.44, 7.38, 7.32, 7.26, 7.2, 7.140000000000001, 7.08, 7.0200000000000005, -4.98, -5.04, -5.1000000000000005, -5.16, -5.22, -5.28, -5.34, -5.4, -5.46, 7.98, 7.92, 7.86, 7.8, 7.74, 7.68, 7.62, 7.5600000000000005, 7.5, -5.04, -5.1000000000000005, -5.16, -5.22, -5.28, -5.34, -5.4, -5.46, -5.5200000000000005, -5.58, -5.64, -5.7, -5.76, 8.46, 8.4, 8.34, 8.28, 8.22, 8.16, 8.1, 8.040000000000001, 7.98, 7.92, 7.86, 7.8, 7.74, 7.68, 7.62, -5.22, -5.28, -5.34, -5.4, -5.46, -5.5200000000000005, -5.58, -5.64, -5.7, -5.76, -5.82, -5.88, -5.94, -6.0, -6.0600000000000005, -6.12, -6.18, -6.24, -6.3, 8.88, 8.82, 8.76, 8.700000000000001, 8.64, 8.58, 8.52, 8.46, 8.4, 8.34, 8.28, 8.22, 8.16, -5.64, -5.7, -5.76, -5.82, -5.88, -5.94, -6.0, -6.0600000000000005, -6.12, -6.18, -6.24, -6.3, -6.36, -6.42, 8.88, 8.82, 8.76, 8.52, 8.46, -6.0600000000000005, -6.12, -6.18, -6.24, -6.3, -6.36, -6.42, -5.16, -5.22, -5.28, -5.34, -5.4, -5.46, -5.5200000000000005, -5.58, -5.64, -4.92, -4.98, -5.04, -5.1000000000000005, -5.16, -5.22, -5.28, -5.34, -5.4, -5.46, -5.5200000000000005, -5.58, -5.64, -4.68, -4.74, -4.8, -4.86, -4.92, -4.98, -5.04, -5.1000000000000005, -5.16, -5.22, -5.28, -5.34, -5.4, -5.46, -4.32, -4.38, -4.44, -4.5, -4.5600000000000005, -4.62, -4.68, -4.74, -4.8, -4.0200000000000005, -4.08, -4.14, -4.2, -4.26, -4.32, -4.38, -4.44, -4.5, -4.5600000000000005, -4.62, -4.68, -3.84, -3.9, -3.96, -4.0200000000000005, -4.08, -4.14, -4.2, -4.26, -4.32, -4.38, -4.44, -4.5, 9.0, 8.94, 8.88, 8.82, 8.76, 8.700000000000001, 8.64, 8.58, 8.52, 8.46, -3.54, -3.6, -3.66, -3.72, -3.7800000000000002, -3.84, -3.9, -3.96, -4.0200000000000005, -4.08, 9.0, 8.94, 8.88, 8.82, 8.76, 8.700000000000001, 8.64, 8.58, 8.52, 8.46, 7.92, 7.86, 7.8, 7.74, 7.68, 7.62, 7.5600000000000005, 7.5, -3.3000000000000003, -3.36, -3.42, -3.48, -3.54, -3.6, -3.66, -3.72, -3.7800000000000002, -3.84, 7.92, 7.86, 7.8, 7.74, 7.68, 7.62, 7.5600000000000005, 7.5, 7.44, 7.38, 7.32, 7.26, 7.2, 7.140000000000001, 7.08, 7.0200000000000005, 6.96, 6.9, 6.84, 6.78, -2.94, -3.0, -3.06, -3.12, -3.18, -3.24, -3.3000000000000003, -3.36, -3.42, -3.48, -3.54, -3.6, 7.74, 7.68, 7.62, 7.5600000000000005, 7.5, 7.44, 7.38, 7.32, 7.26, 7.2, 7.140000000000001, 7.08, 7.0200000000000005, 6.96, 6.9, 6.84, 6.78, 6.72, 6.66, 6.6000000000000005, 6.54, 6.48, 6.42, -2.64, -2.7, -2.7600000000000002, -2.82, -2.88, -2.94, -3.0, -3.06, -3.12, -3.18, -3.24, -3.3000000000000003, -3.36, 7.26, 7.2, 7.140000000000001, 7.08, 7.0200000000000005, 6.96, 6.9, 6.84, 6.78, 6.72, 6.66, 6.6000000000000005, 6.54, 6.48, 6.42, 6.36, 6.3, 6.24, 6.18, 6.12, 6.0600000000000005, 6.0, -2.22, -2.2800000000000002, -2.34, -2.4, -2.46, -2.52, -2.58, -2.64, -2.7, -2.7600000000000002, -2.82, -2.88, -2.94, -3.0, -3.06, 6.36, 6.3, 6.24, 6.18, 6.12, 6.0600000000000005, 6.0, 5.94, 5.88, 5.82, 5.76, 5.7, -1.68, -1.74, -1.8, -1.86, -1.92, -1.98, -2.04, -2.1, -2.16, -2.22, -2.2800000000000002, -2.34, -2.4, -2.46, -2.52, -2.58, -2.64, 6.0600000000000005, 6.0, 5.94, 5.88, 5.82, 5.76, 5.7, 5.64, 5.58, 5.5200000000000005, 5.46, 5.4, 5.34, 5.28, 5.22, 5.16, 5.1000000000000005, 5.04, 4.98, -1.44, -1.5, -1.56, -1.62, -1.68, -1.74, -1.8, -1.86, -1.92, -1.98, -2.04, -2.1, -2.16, -2.22, -2.2800000000000002, 5.64, 5.58, 5.5200000000000005, 5.46, 5.4, 5.34, 5.28, 5.22, 5.16, 5.1000000000000005, 5.04, 4.98, 4.92, 4.86, 4.8, 4.74, 4.68, 4.62, 4.5600000000000005, 4.5, 4.44, 4.38, 4.32, -1.3800000000000001, -1.44, -1.5, -1.56, -1.62, -1.68, -1.74, -1.8, -1.86, -6.0600000000000005, -6.12, -6.18, 5.34, 5.28, 5.22, 5.16, 5.1000000000000005, 5.04, 4.98, 4.92, 4.86, 4.8, 4.74, 4.68, 4.62, 4.5600000000000005, 4.5, 4.44, 4.38, 4.32, 4.26, 4.2, 4.14, 4.08, 4.0200000000000005, 3.96, -1.1400000000000001, -1.2, -1.26, -1.32, -1.3800000000000001, -1.44, -1.5, -6.0, -6.0600000000000005, -6.12, -6.18, 4.86, 4.8, 4.74, 4.68, 4.62, 4.5600000000000005, 4.5, 4.44, 4.38, 4.32, 4.26, 4.2, 4.14, 4.08, 4.0200000000000005, 3.96, 3.9, 3.84, 3.7800000000000002, 3.72, -0.42, -0.48, -0.54, -0.6, -0.66, -0.72, -0.78, -0.84, -0.9, -0.96, -1.02, -1.08, -1.1400000000000001, -1.2, -1.26, -1.32, -5.94, -6.0, -6.0600000000000005, -6.12, 4.2, 4.14, 4.08, 4.0200000000000005, 3.96, 3.9, 3.84, 3.7800000000000002, 3.72, 3.66, 3.6, 3.54, 3.48, 3.42, 3.36, 3.3000000000000003, 3.24, 3.18, 3.12, 3.06, 3.0, 2.94, 2.88, 2.82, 2.7600000000000002, 2.7, 2.64, 2.58, 0.78, 0.72, 0.66, 0.6, 0.54, 0.48, 0.42, 0.36, 0.3, 0.24, 0.18, 0.12, 0.06, -0.0, -0.06, -0.12, -0.18, -0.24, -0.3, -0.36, -0.42, -0.48, -0.54, -0.6, -0.66, -0.72, -0.78, -0.84, -0.9, -0.96, -1.02, -1.08, -1.1400000000000001, -5.94, -6.0, 3.9, 3.84, 3.7800000000000002, 3.72, 3.66, 3.6, 3.54, 3.48, 3.42, 3.36, 3.3000000000000003, 3.24, 3.18, 3.12, 3.06, 3.0, 2.94, 2.88, 2.82, 2.7600000000000002, 2.7, 2.64, 2.58, 2.52, 2.46, 2.4, 2.34, 2.2800000000000002, 2.22, 2.16, 2.1, 2.04, 1.98, 1.92, 1.86, 1.8, 1.74, 1.68, 1.62, 1.56, 1.5, 1.44, 1.3800000000000001, 1.32, 1.26, 1.2, 1.1400000000000001, 1.08, 1.02, 0.96, 0.9, 0.84, 0.78, 0.72, 0.66, 0.6, 0.54, 0.48, 0.42, 0.36, 0.3, 0.24, 0.18, 0.12, 0.06, -0.0, -0.06, -0.12, -0.18, -0.24, -0.3, -0.36, -0.42, -0.48, -0.54, -0.6, -0.66, -0.72, -0.78, -0.84, -0.9, -0.96, -5.7, -5.76, -5.82, 3.84, 3.7800000000000002, 3.72, 3.66, 3.6, 3.54, 3.48, 3.42, 3.36, 3.3000000000000003, 3.24, 3.18, 3.12, 3.06, 3.0, 2.94, 2.88, 2.82, 2.7600000000000002, 2.7, 2.64, 2.58, 2.52, 2.46, 2.4, 2.34, 2.2800000000000002, 2.22, 2.16, 2.1, 2.04, 1.98, 1.92, 1.86, 1.8, 1.74, 1.68, 1.62, 1.56, 1.5, 1.44, 1.3800000000000001, 1.32, 1.26, 1.2, 1.1400000000000001, 1.08, 1.02, 0.96, 0.9, 0.84, 0.78, 0.72, 0.66, 0.6, 0.54, 0.48, 0.42, 0.36, 0.3, 0.24, 0.18, 0.12, 0.06, -0.0, -0.06, -0.12, -0.18, -5.64, -5.7, -5.76, -5.82, 2.4, 2.34, 2.2800000000000002, 2.22, 2.16, 2.1, 2.04, 1.98, 1.92, 1.86, -5.5200000000000005, -5.58, -5.64, -5.7, -5.34, -5.4, -5.46, -5.5200000000000005, -5.58, -5.22, -5.28, -5.34, -5.4, -5.46, -5.5200000000000005, -5.16, -5.22, -5.28, -5.34, -5.04, -5.1000000000000005, -5.16, -5.22, -5.28, -4.92, -4.98, -5.04, -5.1000000000000005, -5.16, -5.22, -4.92, -4.98, -5.04, -5.1000000000000005, -5.16, -4.74, -4.8, -4.86, -4.92, -4.98, -4.74, -4.8, -4.86, -4.92, -4.62, -4.68, -4.74, -4.8, -4.5, -4.5600000000000005, -4.62, -4.68, -4.74, -6.36, -6.42, -4.44, -4.5, -4.5600000000000005, -4.62, -4.68, -5.58, -5.64, -5.7, -6.36, -6.42]}]
  in  "Make WPT":bool
  in  "mission auto":bool=TRUE
  # "Traffic Signal"
  # "Sign Detection"
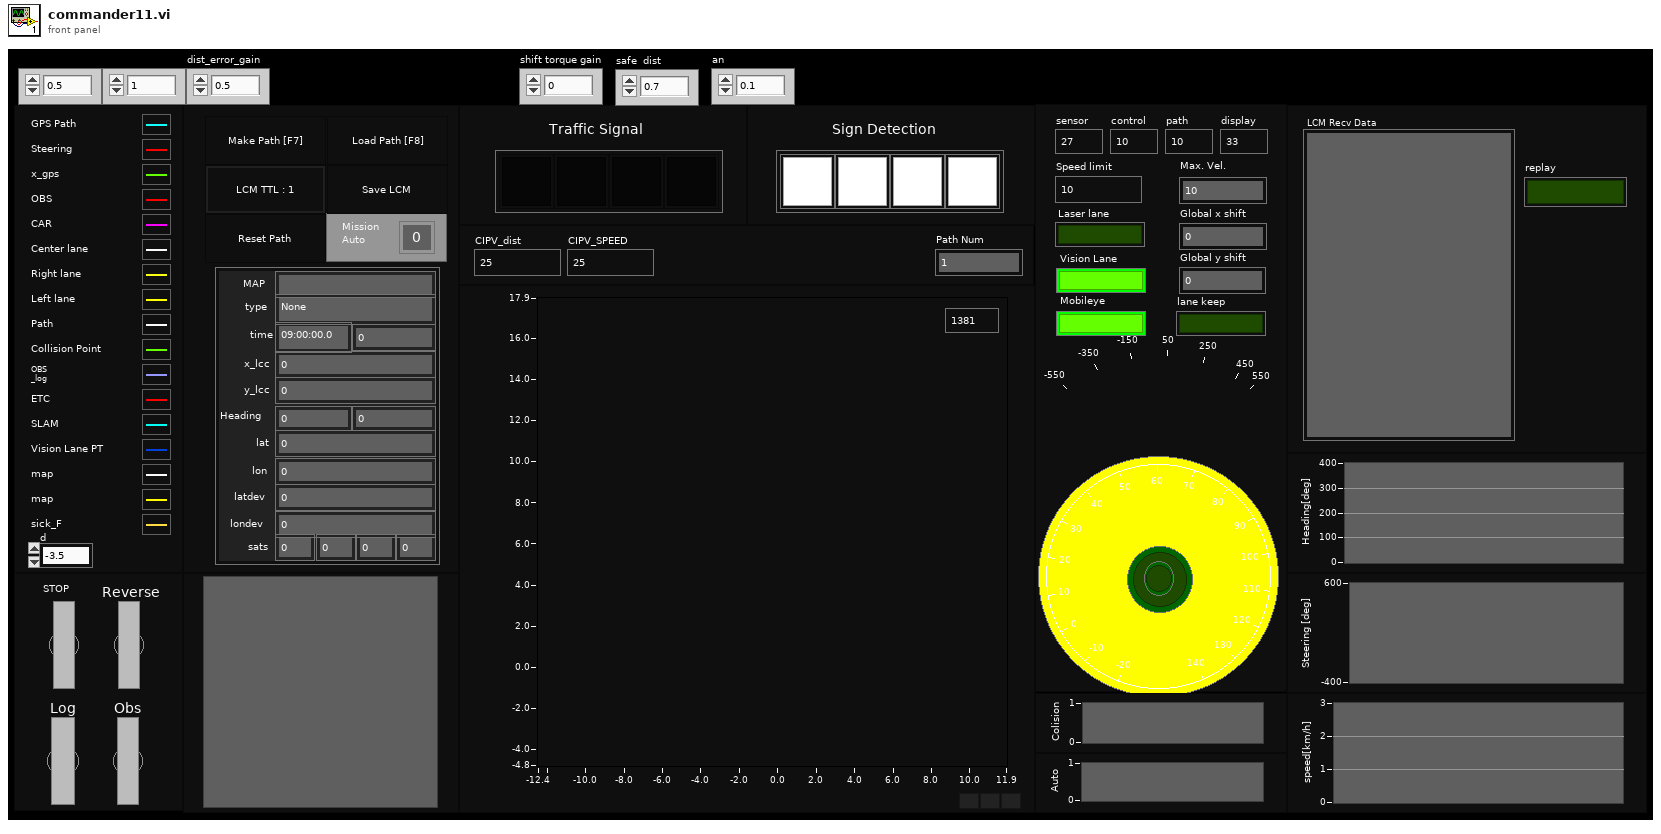
[diagram p1: front panel]
types:
  T1 = cluster{"type":string, "x_lcc":dbl, "y_lcc":dbl, "latdev":sgl, "londev":sgl, "sats":u8, "gps_l1_ranges":u8, "gps_l1_mask_ranges":u8, "gps_l2_mask_ranges":u8, "Heading":dbl, "lon":sgl, "lat":sgl, "time":string, "hgps":dbl, "lag":dbl, "MAP":string}
  T2 = cluster{"VS_des":dbl, "VS_can":dbl, "VS_des":dbl}
  T3 = enum8{"Enabled", "Disabled", "Disabled and Grayed Out"}
  T4 = typedef "Dynamixel Pro Driver.lvlib/Write Select Pro.ctl" = enum16{"ID", "Baud Rate", "Return Delay Time", "Operating mode", "Homing offset", "Moving threshold", "Temperature limit", "Max Voltage Limit", "Min Voltage Limit", "acceleration Limit", "Torque Limit", "Velocity Limit", "Max Position Limit", "Min Position Limit", "External Port Mode 1", "External Port Mode 2", "External Port Mode 3", "External Port Mode 4", "Shutdown", "Torque Enable", "LED RED", "LED GREEN", "LED BLUE", "Velocity I Gain", "Velocity P Gain", "Position P Gain", "Goal Position", "Goal Velocity", "Goal Torque", "Goal Acceleration", "External Port Data 1", "External Port Data 2", "External Port Data 3", "External Port Data 4", "Status Return Level"}
  T5 = typedef "Dynamixel Pro Driver.lvlib/Baudrate Selector.ctl" = enum16{"2400", "57600", "115200", "1000000", "2000000", "3000000", "4000000", "4500000", "10500000"}
  T6 = cluster{"Steer_input":dbl, "Steer_output":dbl, "VS_des":dbl, "VS_can":dbl, "heading":dbl, "auto":bool, "run":bool, "x":dbl, "y":dbl, "slam_y":dbl, "slam_x":dbl, "slam_heading":dbl}
  T7 = cluster{"hash":i64, "sys time":i64, "signal":i32, "sign":i32, "pedestrian":bool, "flag car":bool, "distance":dbl}
  T8 = typedef "imagedata.ctl" = cluster{"image type":i32, "image depth":i32, "image":u8[], "mask":u8[], "colors":u32[], "Rectangle":cluster{"left":i16, "top":i16, "right":i16, "bottom":i16}}
  T9 = cluster{"hash":i64, "sys time":i64, "status":i32, "TS_num":i32, "TS_type":i32[], "TS_loc_x":dbl[], "TS_loc_y":dbl[]}
  T10 = cluster{"hash":i64, "sys time":i64, "s_lat":dbl, "s_lon":dbl, "d_lat":dbl, "d_lon":dbl, "Message":i64}
  T11 = cluster{"beep":bool, "duration (msec)":u32, "frequency (Hz)":u32}
  T12 = cluster{"identifier":u32, "timestamp":timestamp, "payload":u8[]}
  T13 = enum32{"Namyang", "Hyundai", "KAIST", "Ajou", "Munji", "Airforce", "Car", "KATRI", "Samsung", "Coex", "Gwangnaru", "Inje", "sinjin", "NAVER"}
  T14 = cluster{"hash":i64, "sys time":i64, "size":i32, "data":u8[]}
  T15 = cluster{"Minimum":dbl, "Minimum":dbl, "Minimum":dbl, "Minimum":dbl, "Minimum":dbl}
  T16 = cluster{"hash":i64, "sys time":i64, "time":dbl, "x":dbl, "y":dbl, "h":dbl, "numSV":i32, "postype":i32, "lag":i32, "hordev":dbl, "lat":dbl, "lon":dbl, "hgt":dbl, "map_idx":i32}
  T17 = enum16{"Velodyne 16", "Velodyne 32", "Velodyne 64"}
  T18 = cluster{"hash":i64, "sys time":i64, "size":i64, "x":dbl[], "y":dbl[], "point_flag":i32[]}
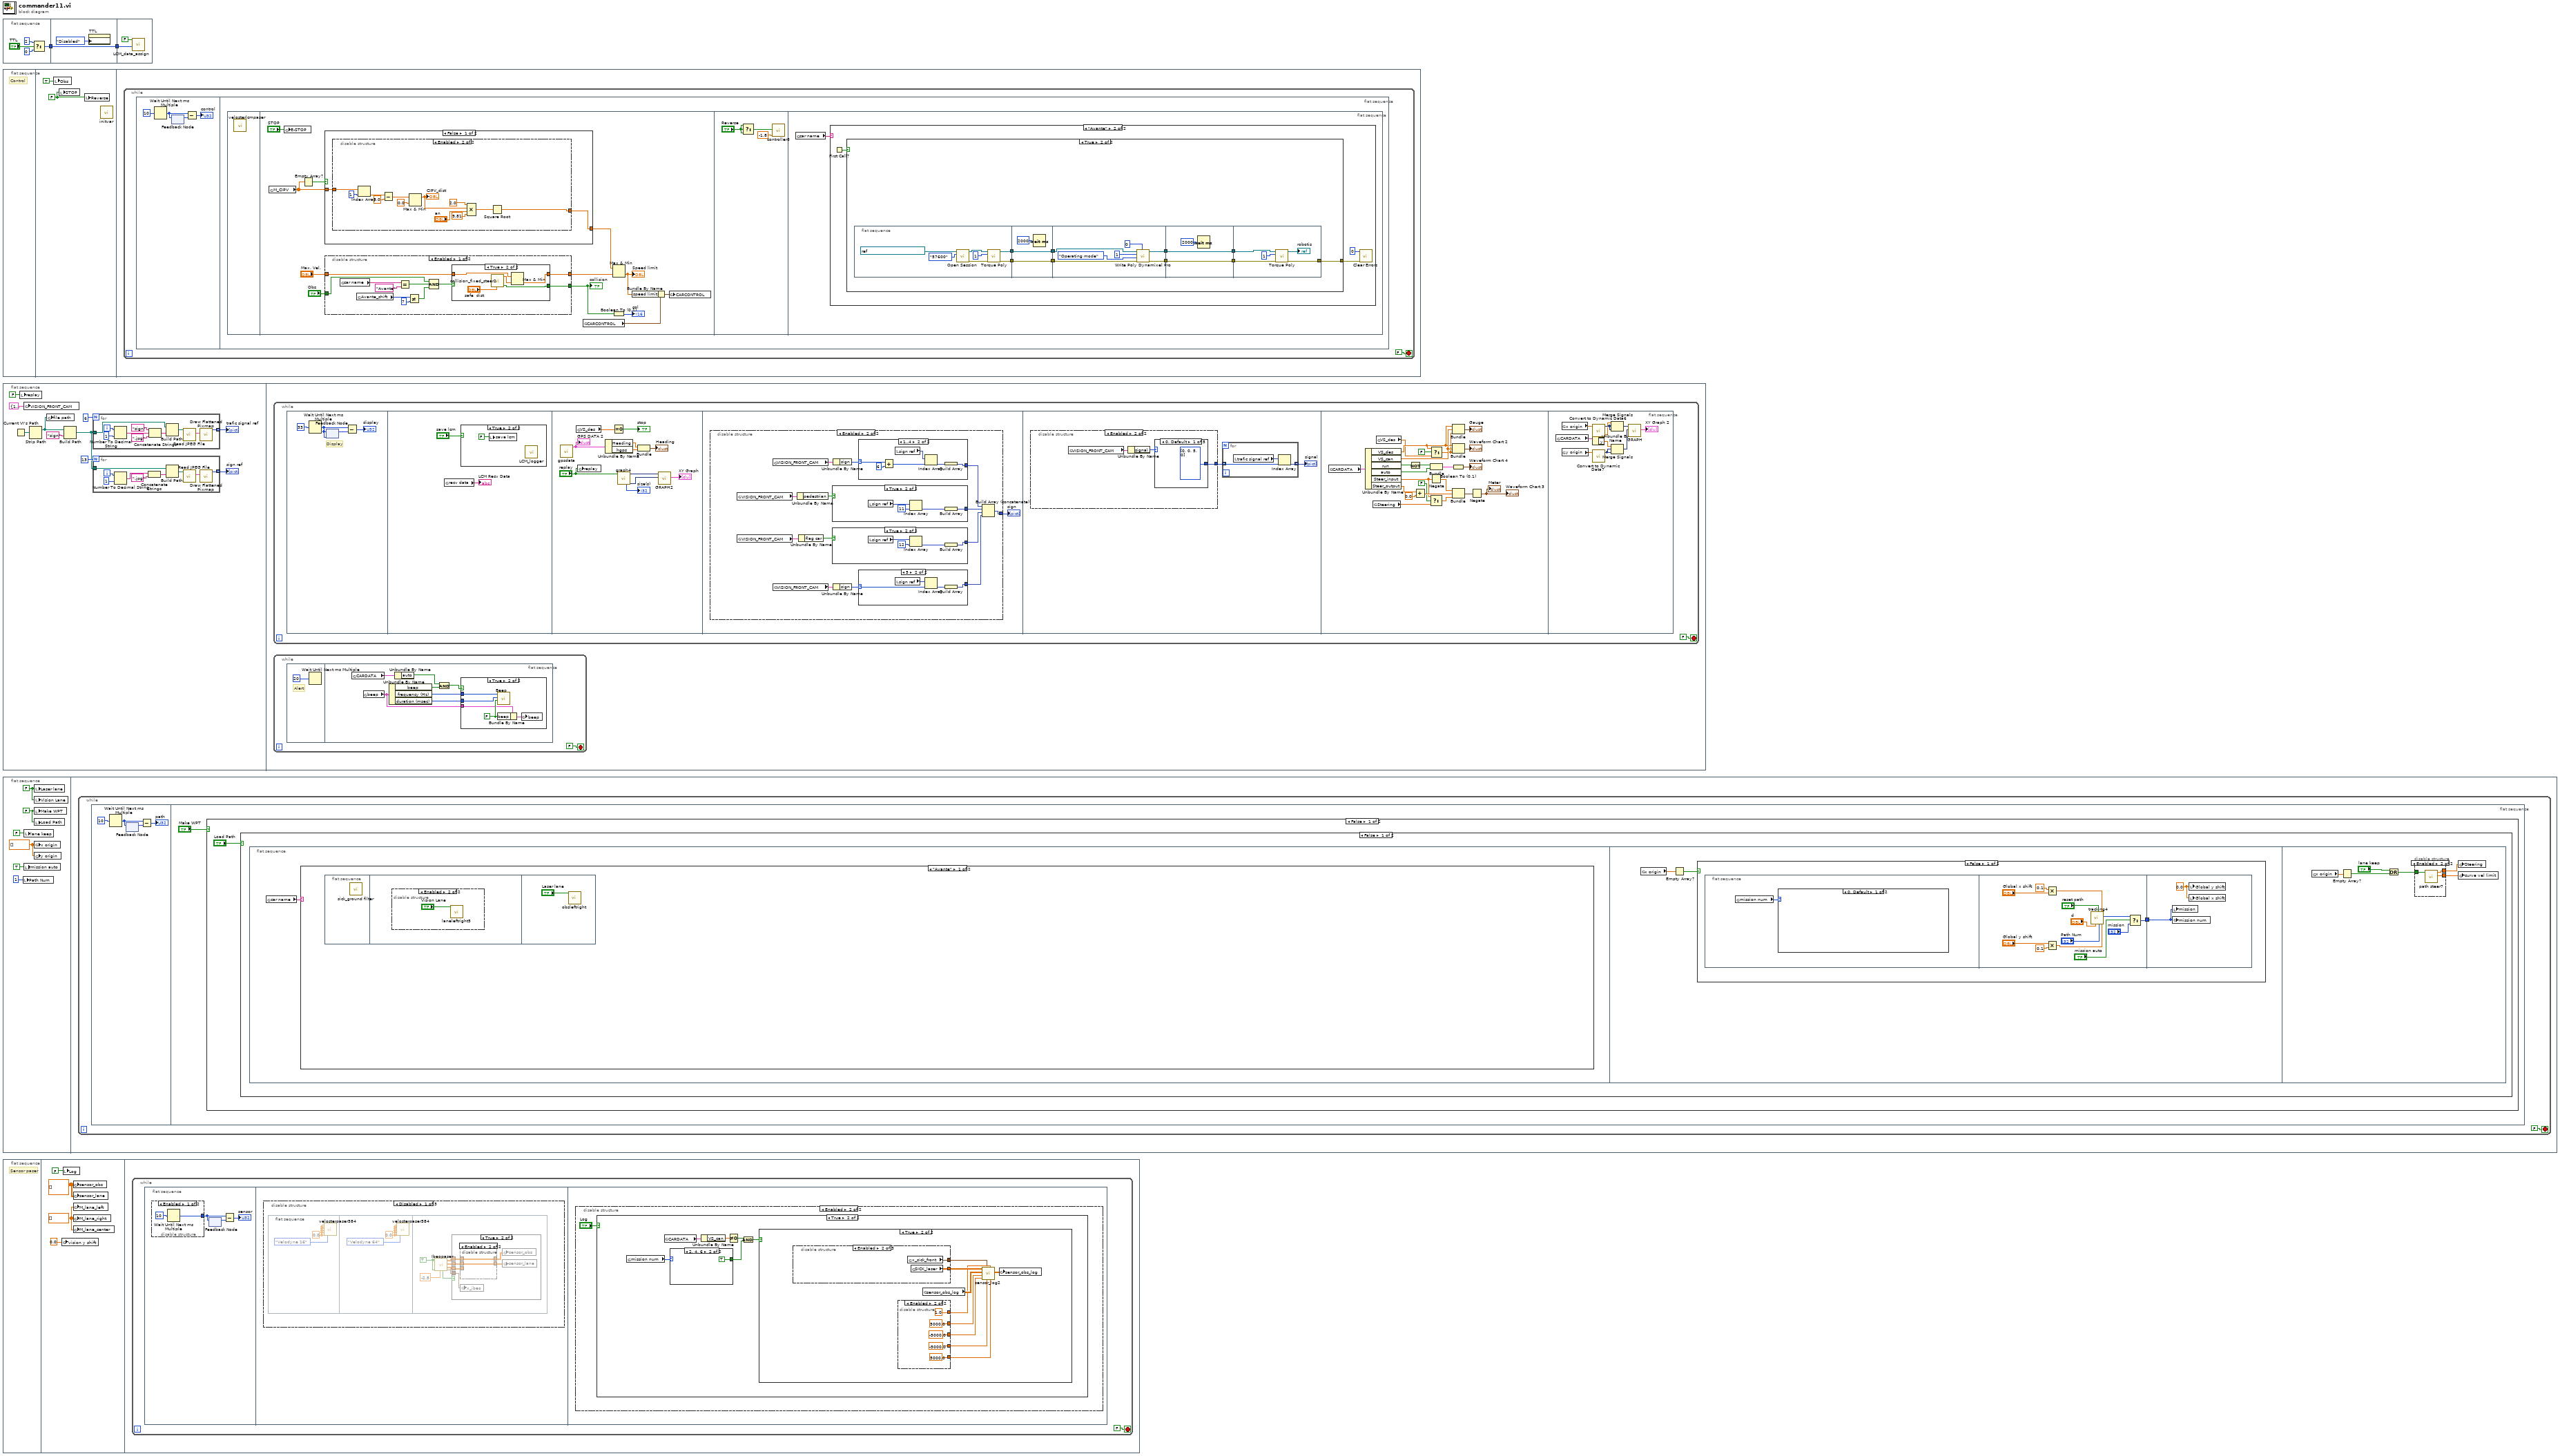
[diagram p0: block diagram]
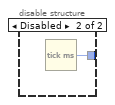
[diagram p2: hidden frame]
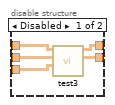
[diagram p4: hidden frame]
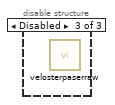
[diagram p6: hidden frame]
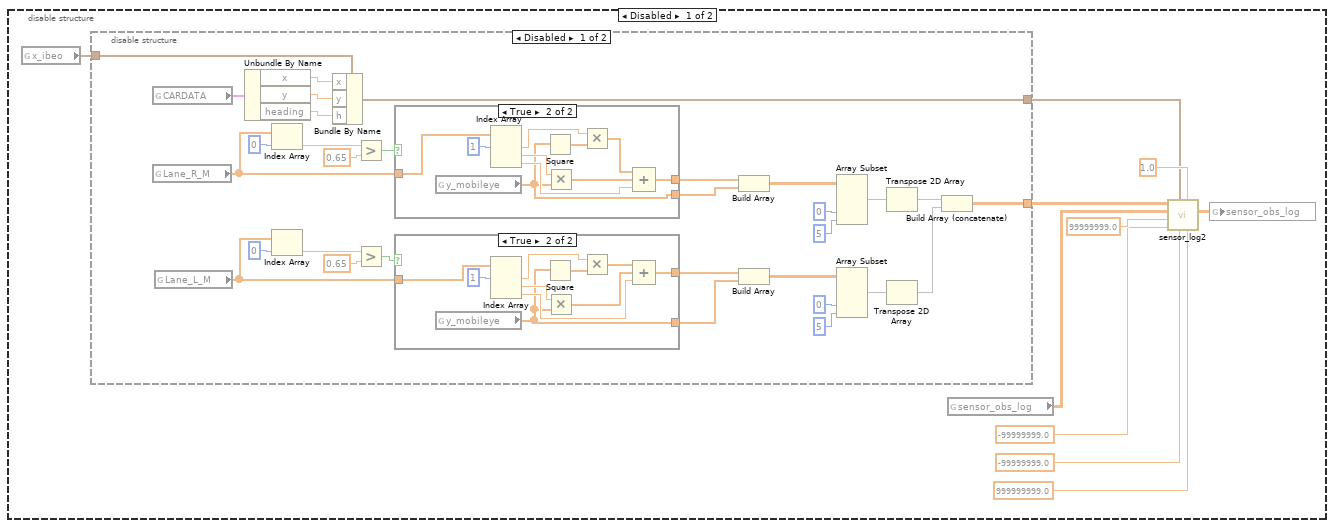
[diagram p7: hidden frame]
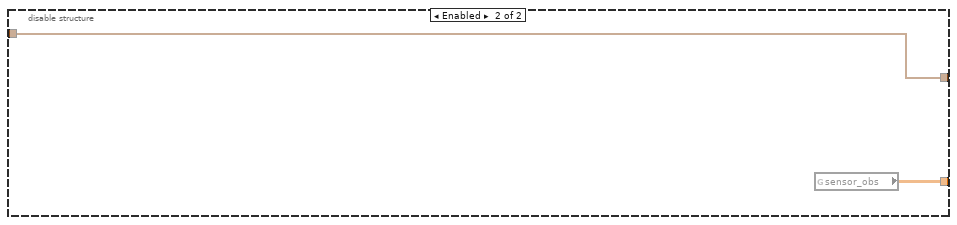
[diagram p10: hidden frame]
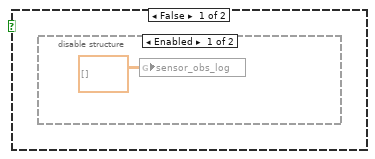
[diagram p11: hidden frame]
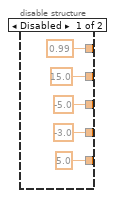
[diagram p15: hidden frame]
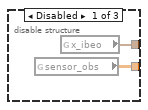
[diagram p16: hidden frame]
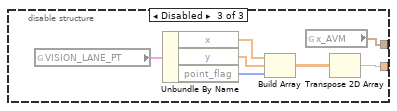
[diagram p17: hidden frame]
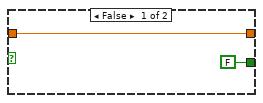
[diagram p18: hidden frame]
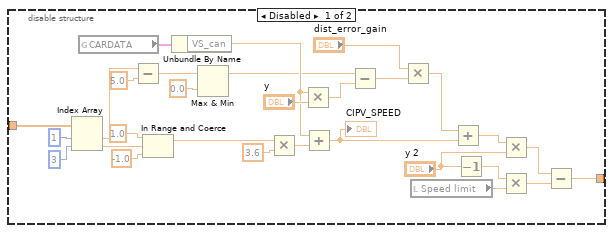
[diagram p20: hidden frame]
diagram:
  n1 = flat-sequence {
    tunnel: [w3] -> w1
    tunnel: [w7] -> w2
    tunnel: w1 -> [w7]
    tunnel: w2 -> [w9]
    frame #0 {
      n2 = Select(t=u16 2 ("time-to-live"), s="TTL", f=u16 0 ("time-to-live")) -> (s? t:f=w3:u16)
    }
    frame #1 {
      n3 = property on="TTL" class="Bool (strict)"("DisabledEnum"=T3."Disabled" ("Disabled")) -> ()  [unwired: 2 in, 2 out]
    }
    frame #2 {
      n4 = call "LCM_data_assign.vi"("time-to-live"=w9, "velodyne enable"=FALSE) -> ()  [unwired: 10 in]
    }
  }
  n5 = flat-sequence {
    frame #0 {
      # "Control"
    }
    frame #1 {
      w12 = FALSE ("LCM")
      n6 = local write "Obs"(TRUE ("obs")) -> ()
      n7 = local write "STOP"(w12) -> ()
      n8 = local write "Reverse"(w12) -> ()
      n9 = call "initvar.vi"() -> ()  [unwired: 12 in]
    }
    frame #2 {
      n10 = while {
        stop <- FALSE ("Loop 1") stop-if-true
        n11 = flat-sequence {
          frame #0 {
            n12 = Wait Until Next ms Multiple(millisecond multiple=u32 10 ("milliseconds to wait")) -> (millisecond timer value=w14:u32)
            n13 = feedback #1() -> (w15:u32)  [unwired: 1 in]
            n14 = feedback-in #1(w14) -> ()
            n15 = Subtract(x=w14, y=w15) -> (x-y=→"control":u32)
          }
          frame #1 {
            n16 = flat-sequence {
              frame #0 {
                n17 = call "velosterlcmpaser.vi"() -> ()  [unwired: 11 in, 1 out]
              }
              frame #1 {
                n18 = global read "G_SEN.vi" "M_CIPV"() -> (w22:dbl[])
                n19 = global write "G_ALL.vi" "E-STOP"("STOP") -> ()
                n20 = Empty Array?(array=w22) -> (empty?=w23:bool)
                n21 = case shown="False" w23 {
                  tunnel: w22 -> [w50 _]
                  tunnel: [w49 w93] -> w19
                  frame False {
                    n22 = disable-structure shown="Enabled" {
                      disable-tunnel: w50 -> [w79 w86]
                      disable-tunnel: [w62 w82] -> w49
                      frame Disabled {
                        n23 = Index Array(array=w79, index #1=1 ("index"), index #2=3 ("index")) -> (element #1=w57:dbl, element #2=w61:dbl)
                        n24 = global read "G_ALL.vi" "CARDATA"() -> (w77:T6)
                        n25 = Subtract(x=w57, y=5.0) -> (x-y=w55:dbl)
                        n26 = In Range and Coerce(upper limit=1.0, x=w61, lower limit=-1.0) -> (coerced(x)=w58:dbl)  [unwired: 1 out]
                        n27 = Unbundle By Name(w77) -> ("VS_can"=w53:dbl)
                        n28 = Max & Min(x=w55, y=0.0) -> (max(x,y)=w52:dbl)  [unwired: 1 out]
                        n29 = Multiply(x=w58, y=3.6) -> (x*y=w71:dbl)
                        n30 = Multiply(x=w53, y="y") -> (x*y=w69:dbl)
                        n31 = Add(x=w53, y=w71) -> (x+y=w51:dbl)
                        "CIPV_SPEED" <- w51
                        n32 = Subtract(x=w52, y=w69) -> (x-y=w72:dbl)
                        n33 = Multiply(x="dist_error_gain", y=w72) -> (x*y=w74:dbl)
                        n34 = local read "Speed limit"() -> (w65:dbl)
                        n35 = Add(x=w74, y=w51) -> (x+y=w68:dbl)
                        n36 = Decrement(x="y 2") -> (x-1=w66:dbl)
                        n37 = Multiply(x=w68, y="y 2") -> (x*y=w63:dbl)
                        n38 = Multiply(x=w66, y=w65) -> (x*y=w64:dbl)
                        n39 = Subtract(x=w63, y=w64) -> (x-y=w62:dbl)
                      }
                      frame Enabled {
                        n40 = Index Array(array=w86, index=1) -> (element=w90:dbl)
                        n41 = Subtract(x=w90, y=5.0) -> (x-y=w88:dbl)
                        n42 = Max & Min(x=w88, y=0.0) -> (max(x,y)=w80:dbl)  [unwired: 1 out]
                        "CIPV_dist" <- w80
                        n43 = Compound Arithmetic op=MULTIPLY(2.0 ("value"), w80, "an", 9.81 ("value")) -> (w83:dbl)
                        n44 = Square Root(x=w83) -> (sqrt(x)=w82:dbl)
                      }
                    }
                  }
                  frame True {
                    n45 = local read "Speed limit"() -> (w94:dbl)
                    n46 = Add(x=w94, y=3.0) -> (x+y=w93:dbl)
                  }
                }
                n47 = disable-structure shown="Enabled" {
                  disable-tunnel: "Max. Vel." -> [w31 w48]
                  disable-tunnel: [w40 _] -> w27
                  disable-tunnel: [w30 w48] -> w18
                  disable-tunnel: "Obs" -> [w35 _]
                  frame Enabled {
                    n48 = global read "G_LCM.vi" "car name"() -> (w36:string)
                    n49 = global read "G_ALL.vi" "Avante_shift"() -> (w38:u8)
                    n50 = Equal?(x=w36, y="Avante") -> (x = y?=w34:bool)
                    n51 = Not Equal?(x=w38, y=u8 7) -> (x != y?=w33:bool)
                    n52 = Compound Arithmetic op=AND(w35, w34, w33) -> (w32:bool)
                    n53 = case shown="True" w32 {
                      tunnel: [FALSE ("collision") w46] -> w40
                      tunnel: [w41 w43] -> w30
                      tunnel: w31 -> [w41 w44]
                      frame False {
                      }
                      frame True {
                        n54 = call "collision_fixed_steer2.vi"("safe  dist"="safe  dist") -> ("collision"=w46:bool, "speed limit"=w45:dbl)  [unwired: 8 in, 1 out]
                        n55 = Max & Min(x=w44, y=w45) -> (min(x,y)=w43:dbl)  [unwired: 1 out]
                      }
                    }
                  }
                  frame Disabled {
                  }
                }
                "collision" <- w27
                n56 = global read "G_ALL.vi" "CARCONTROL"() -> (w25:cluster{"speed path":dbl, "speed limit":dbl})
                n57 = Boolean To (0,1)(Boolean=w27) -> (0, 1=→"col":i16)
                n58 = Max & Min(x=w19, y=w18) -> (min(x,y)=w21:dbl)  [unwired: 1 out]
                "Speed limit" <- w21
                n59 = Bundle By Name(cluster=w25, "speed limit"=w21) -> (w24:cluster{"speed path":dbl, "speed limit":dbl})
                n60 = global write "G_ALL.vi" "CARCONTROL"(w24) -> ()
              }
              frame #2 {
                n61 = Select(t="Reverse", s="Reverse", f="Reverse") -> (s? t:f=w96:bool)
                n62 = call "controller8.vi"("Neg max speed"=-1.8, "reverse"=w96) -> ()  [unwired: 10 in]
              }
              frame #3 {
                n63 = global read "G_LCM.vi" "car name"() -> (w98:string)
                n64 = case shown="\"Avante\"" w98 {
                  frame Default {
                  }
                  frame "Avante" {
                    n65 = First Call?() -> (First Call?: T/F=w101:bool)
                    n66 = case shown="True" w101 {
                      tunnel: [w121 w127] -> w100
                      frame False {
                        n67 = global read "G_ALL.vi" "Avante_shift"() -> (w110:u8)
                        n68 = case shown="5, Default" w110 {
                          tunnel: [0 -1] -> w108
                          frame 5, Default {
                          }
                          frame 0, 6, 7 {
                          }
                        }
                        n69 = case shown="7, Default" w110 {
                          tunnel: [0 1 -1] -> w107
                          frame 7, Default {
                          }
                          frame 5, 6 {
                          }
                          frame 0 {
                          }
                        }
                        n70 = global read "G_ALL.vi" "VS_des"() -> (w102:dbl)
                        n71 = global read "G_ALL.vi" "CARDATA"() -> (w114:T6)
                        n72 = Greater Or Equal To 0?(x=w102) -> (x >= 0?=w109:bool)
                        n73 = Unbundle By Name(w114) -> ("auto"=w112:bool, "VS_can"=w113:dbl)
                        n74 = Select(t=w108, s=w109, f=w107) -> (s? t:f=w106:i32)
                        n75 = Negate(x=w106) -> (-x=w105:i32)
                        n76 = Equal To 0?(x=w113) -> (x = 0?=w111:bool)
                        n77 = Multiply(x="shift torque gain", y=w105) -> (x*y=w116:i32)
                        n78 = And(x=w112, y=w111) -> (x .and. y?=w120:bool)
                        n79 = local read "robotis"() -> (w104:refnum<visa-resource-name>)
                        n80 = Select(t=w116, s=w120, f=0) -> (s? t:f=w117:i32)
                        n81 = call-poly <vilib>:"Write Poly Dynamixel Pro.vi"("Value"=w117, "Operation"=Write_Select_Pro."Goal Torque", "ID"=u8 1, "VISA Refnum in"=w104) -> ("error out"=w121:errorcluster)  [unwired: 6 in, 1 out]
                      }
                      frame True {
                        n82 = flat-sequence {
                          tunnel: [w138] -> w135
                          tunnel: [w137] -> w134
                          tunnel: [w145] -> w133
                          tunnel: w135 -> [w145]
                          tunnel: [w144] -> w132
                          tunnel: w134 -> [w144]
                          tunnel: [w149] -> w131
                          tunnel: w133 -> [w151]
                          tunnel: w132 -> [w150]
                          tunnel: [w148] -> w130
                          tunnel: w131 -> [w155]
                          tunnel: [w155] -> w129
                          tunnel: [w154] -> w128
                          tunnel: w130 -> [w154]
                          tunnel: [w158] -> w127
                          tunnel: w129 -> [w160]
                          tunnel: w128 -> [w159]
                          frame #0 {
                            n83 = call <vilib>:"Open Session.vi"("Baud Rate"=Baudrate_Selector."57600", "VISA resource name"=refnum<visa-resource-name> "COM5") -> ("error out"=w141:errorcluster, "VISA Refnum out"=w142:refnum<visa-resource-name>)  [unwired: 8 in]
                            n84 = call-poly <vilib>:"Torque Poly.vi"("error in (no error)"=w141, "ID"=u8 1, "VISA Refnum in"=w142) -> ("error out"=w137:errorcluster, "VISA Refnum out"=w138:refnum<visa-resource-name>)  [unwired: 7 in]
                          }
                          frame #1 {
                            n85 = Wait (ms)(milliseconds to wait=u32 2000) -> ()  [unwired: 1 out]
                          }
                          frame #2 {
                            n86 = call-poly <vilib>:"Write Poly Dynamixel Pro.vi"("Value"=0, "error in (no error)"=w150, "Operation"=Write_Select_Pro."Operating mode", "ID"=u8 1, "VISA Refnum in"=w151) -> ("error out"=w148:errorcluster, "VISA Refnum out"=w149:refnum<visa-resource-name>)  [unwired: 5 in]
                          }
                          frame #3 {
                            n87 = Wait (ms)(milliseconds to wait=u32 2000) -> ()  [unwired: 1 out]
                          }
                          frame #4 {
                            n88 = call-poly <vilib>:"Torque Poly.vi"("error in (no error)"=w159, "ID"=u8 1, "VISA Refnum in"=w160) -> ("error out"=w158:errorcluster, "VISA Refnum out"=→"robotis":refnum<visa-resource-name>)  [unwired: 7 in]
                          }
                        }
                      }
                    }
                    n89 = call <vilib>:"Clear Errors.vi"("error in (no error)"=w100, "specific error code to clear (0: all)"=0) -> ()  [unwired: 4 in, 2 out]
                  }
                }
              }
            }
          }
        }
      }
    }
  }
  n90 = flat-sequence {
    frame #0 {
      n91 = Current VI's Path() -> (path=w169:path)
      n92 = local write "replay"(FALSE ("replay")) -> ()
      n93 = global write "G_LCM.vi" "VISION_FRONT_CAM"(T7 {"hash"=1386151893206175709, "sys time"=1, "signal"=1, "sign"=3, "pedestrian"=TRUE, "flag car"=TRUE, "distance"=0.0} ("VISION_FRONT_CAM")) -> ()
      n94 = Strip Path(path=w169) -> (stripped path=w162:path)  [unwired: 1 out]
      n95 = global write "G_ALL.vi" "file path"(w162) -> ()
      n96 = Build Path(base path=w162, name or relative path="sign") -> (appended path=w163:path)
      n97 = for {
        N: 6 -> [_]
        tunnel: [w179] -> w165 mode=indexing
        tunnel: w163 -> [w174]
        i -> [w178]
        n98 = Number To Decimal String(number=w178, width (-)=i16 1) -> (decimal integer string=w176:string)
        n99 = Concatenate Strings("sign" ("string"), w176, ".jpg") -> (w173:string)
        n100 = Build Path(base path=w174, name or relative path=w173) -> (appended path=w172:path)
        n101 = call <vilib>:"Read JPEG File.vi"("path to JPEG file"=w172) -> ("image data"=w180:T8)  [unwired: 8 in, 2 out]
        n102 = call <vilib>:"Draw Flattened Pixmap.vi"("image data"=w180) -> ("new picture"=w179:picture)  [unwired: 8 in]
      }
      "trafic signal ref" <- w165
      n103 = for {
        N: 13 -> [_]
        tunnel: [w188] -> w166 mode=indexing
        tunnel: w163 -> [w183]
        i -> [w187]
        n104 = Number To Decimal String(number=w187, width (-)=i16 1) -> (decimal integer string=w185:string)
        n105 = Concatenate Strings(w185, ".jpg") -> (w182:string)
        n106 = Build Path(base path=w183, name or relative path=w182) -> (appended path=w181:path)
        n107 = call <vilib>:"Read JPEG File.vi"("path to JPEG file"=w181) -> ("image data"=w189:T8)  [unwired: 8 in, 2 out]
        n108 = call <vilib>:"Draw Flattened Pixmap.vi"("image data"=w189) -> ("new picture"=w188:picture)  [unwired: 8 in]
      }
      "sign ref" <- w166
    }
    frame #1 {
      n109 = while {
        stop <- FALSE ("Loop 2") stop-if-true
        n110 = flat-sequence {
          frame #0 {
            # "Display"
            n111 = Wait Until Next ms Multiple(millisecond multiple=u32 33 ("milliseconds to wait")) -> (millisecond timer value=w205:u32)
            n112 = feedback #2(w205) -> (w207:u32)
            n113 = feedback-in #2(w205) -> ()
            n114 = Subtract(x=w205, y=w207) -> (x-y=→"display":u32)
          }
          frame #1 {
            n115 = global read "G_LCM.vi" "recv data"() -> (→"LCM Recv Data":string)
            n116 = case shown="True" "save lcm" {
              frame False {
              }
              frame True {
                n117 = local write "save lcm"(FALSE ("save lcm")) -> ()
                n118 = call "LCM_logger.vi"() -> ()  [unwired: 12 in]
              }
            }
          }
          frame #2 {
            n119 = call "gpsdata.vi"() -> ("GPS DATA 2"=w215:T1)  [unwired: 11 in]
            "GPS DATA 2" <- w215
            n120 = global read "G_ALL.vi" "VS_des"() -> (w221:dbl)
            n121 = global write "G_ALL.vi" "replay"("replay") -> ()
            n122 = Unbundle By Name(w215) -> ("Heading"=w213:dbl, "hgps"=w214:dbl)
            n123 = Equal To 0?(x=w221) -> (x = 0?=→"stop":bool)
            n124 = call "graph4.vi"("replay"="replay") -> ("y"=w219:dynamicdata, "x"=w218:dynamicdata, "size(s)"=→"size(s)":i32)  [unwired: 8 in]
            n125 = Bundle("Heading"=w213, "hgps"=w214) -> (→"Heading":cluster{"Heading":dbl, "hgps":dbl})  [unwired: 1 in]
            n126 = call "GRAPH2"("Y Input"=w219, "X Input"=w218) -> ("XY Graph"=→"XY Graph":cluster{"Y":dbl[], "Y":dbl[]}[])  [unwired: 3 in, 6 out]
          }
          frame #3 {
            n127 = disable-structure shown="Enabled" {
              disable-tunnel: [w226 w249] -> w223
              frame Disabled {
                n128 = global read "G_LCM.vi" "EURECAR_VISION"() -> (w227:T9)
                n129 = Unbundle By Name(w227) -> ("TS_num"=w224:i32, "TS_type"=w225:i32[])
                n130 = case shown="0" w224 {
                  tunnel: w225 -> [_ w238]
                  tunnel: [w232 w237] -> w226
                  frame 0 {
                    w234 = 100 ("x")
                    n131 = local read "count"() -> (w235:i32)
                    n132 = Increment(x=w235) -> (x+1=w230:i32)
                    n133 = Max & Min(x=w234, y=w230) -> (min(x,y)=w229:i32)  [unwired: 1 out]
                    n134 = local write "count"(w229) -> ()
                    n135 = Equal?(x=w234, y=w229) -> (x = y?=w228:bool)
                    n136 = local read "sign"() -> (w231:picture[])
                    n137 = Select(t=picture[] [], s=w228, f=w231) -> (s? t:f=w232:picture[])
                  }
                  frame 1, Default {
                    n138 = for {
                      tunnel: w238 -> [w240] mode=indexing
                      tunnel: [w239] -> w237 mode=indexing
                      n139 = local read "sign ref"() -> (w241:picture[])
                      n140 = Index Array(array=w241, index=w240) -> (element=w239:picture)
                    }
                    "count" <- 0 ("Numeric Control")
                  }
                }
              }
              frame Enabled {
                n141 = global read "G_LCM.vi" "VISION_FRONT_CAM"() -> (w248:T7)
                n142 = global read "G_LCM.vi" "VISION_FRONT_CAM"() -> (w247:T7)
                n143 = global read "G_LCM.vi" "VISION_FRONT_CAM"() -> (w253:T7)
                n144 = global read "G_LCM.vi" "VISION_FRONT_CAM"() -> (w244:T7)
                n145 = Unbundle By Name(w248) -> ("pedestrian"=w252:bool)
                n146 = Unbundle By Name(w247) -> ("flag car"=w246:bool)
                n147 = case shown="True" w252 {
                  tunnel: [picture[] [] w266] -> w251
                  frame False {
                  }
                  frame True {
                    n148 = local read "sign ref"() -> (w269:picture[])
                    n149 = Index Array(array=w269, index=11) -> (element=w267:picture)
                    n150 = Build Array(w267) -> (w266:picture[])
                  }
                }
                n151 = case shown="True" w246 {
                  tunnel: [picture[] [] w261] -> w245
                  frame False {
                  }
                  frame True {
                    n152 = local read "sign ref"() -> (w264:picture[])
                    n153 = Index Array(array=w264, index=12) -> (element=w262:picture)
                    n154 = Build Array(w262) -> (w261:picture[])
                  }
                }
                n155 = Unbundle By Name(w253) -> ("sign"=w254:i32)
                n156 = Unbundle By Name(w244) -> ("sign"=w243:i32)
                n157 = case shown="1..4" w254 {
                  selector: w254 -> [_ w275]
                  tunnel: [picture[] [] w271] -> w250
                  frame 0, Default {
                  }
                  frame 1..4 {
                    n158 = Add(x=w275, y=6) -> (x+y=w273:i32)
                    n159 = local read "sign ref"() -> (w276:picture[])
                    n160 = Index Array(array=w276, index=w273) -> (element=w272:picture)
                    n161 = Build Array(w272) -> (w271:picture[])
                  }
                }
                n162 = case shown="5" w243 {
                  selector: w243 -> [_ w258]
                  tunnel: [picture[] [] w256] -> w242
                  frame 0, Default {
                  }
                  frame 5 {
                    n163 = local read "sign ref"() -> (w259:picture[])
                    n164 = Index Array(array=w259, index=w258) -> (element=w257:picture)
                    n165 = Build Array(w257) -> (w256:picture[])
                  }
                }
                n166 = Build Array (concatenate)(w250, w251, w245, w242) -> (w249:picture[])
              }
            }
            "sign" <- w223
          }
          frame #4 {
            n167 = disable-structure shown="Enabled" {
              disable-tunnel: [w285 w293] -> w278
              frame Disabled {
                n168 = global read "G_LCM.vi" "APP_GPS_DATA"() -> (w284:T10)
                n169 = Unbundle By Name(w284) -> ("Message"=w283:i64)
                n170 = Equal To 0?(x=w283) -> (x = 0?=w282:bool)
                n171 = case shown="1" w283 {
                  tunnel: [_ TRUE _ _] -> _
                  tunnel: [i32[] [0, 5, 0, 0] i32[] [1, 5, 0, 0] i32[] [0, 2, 0, 0] i32[] [0, 5, 3, 0]] -> w285
                  frame 0, Default {
                  }
                  frame 1 {
                  }
                  frame 2 {
                  }
                  frame 3 {
                  }
                }
                n172 = Select(t="", s=w282, f="미션중") -> (s? t:f=w279:string)
              }
              frame Enabled {
                n173 = global read "G_LCM.vi" "VISION_FRONT_CAM"() -> (w292:T7)
                n174 = Unbundle By Name(w292) -> ("signal"=w291:i32)
                n175 = case shown="0, Default" w291 {
                  tunnel: [i32[] [0, 0, 5, 0] i32[] [1, 0, 5, 0] i32[] [0, 4, 5, 0] i32[] [0, 0, 2, 0] i32[] [0, 0, 5, 3]] -> w293
                  frame 0, Default {
                  }
                  frame 1 {
                  }
                  frame 2 {
                  }
                  frame 3 {
                  }
                  frame 4 {
                  }
                }
              }
            }
            n176 = for {
              tunnel: w278 -> [w300] mode=indexing
              tunnel: [w299] -> w277 mode=indexing
              n177 = local read "trafic signal ref"() -> (w301:picture[])
              n178 = Index Array(array=w301, index=w300) -> (element=w299:picture)
            }
            "signal" <- w277
          }
          frame #5 {
            n179 = global read "G_ALL.vi" "CARDATA"() -> (w308:T6)
            n180 = Unbundle By Name(w308) -> ("VS_des"=w311:dbl, "VS_can"=w318:dbl, "run"=w316:bool, "auto"=w317:bool, "Steer_input"=w303:dbl, "Steer_output"=w315:dbl)
            n181 = global read "G_ALL.vi" "Steering"() -> (w304:dbl)
            n182 = global read "G_ALL.vi" "VS_des"() -> (w307:dbl)
            n183 = Not(x=w316) -> (.not. x?=w320:bool)
            n184 = Add(x=w315, y=0.0) -> (x+y=w313:dbl)
            n185 = Negate(x=w303) -> (-x=w302:dbl)
            n186 = Select(t=w303, s=FALSE, f=w304) -> (s? t:f=w312:dbl)
            n187 = Select(t=w311, s=FALSE, f=w307) -> (s? t:f=w310:dbl)
            n188 = Bundle(w320, "auto"=w317) -> (w322:cluster{bool, "auto":bool})  [unwired: 1 in]
            n189 = Boolean To (0,1)(Boolean=w322) -> (0, 1=→"Waveform Chart 4":cluster{i16, "auto":i16})
            n190 = Bundle("VS_des"=w311, "VS_can"=w318, "VS_des"=w310) -> (→"Gauge":T2)  [unwired: 1 in]
            n191 = Bundle("VS_des"=w311, "VS_can"=w318, "VS_des"=w310) -> (→"Waveform Chart 2":T2)  [unwired: 1 in]
            n192 = Bundle(w302, w313, "Steering"=w312) -> (w324:cluster{dbl, dbl, "Steering":dbl})  [unwired: 1 in]
            n193 = Negate(x=w324) -> (-x=→"Meter" →"Waveform Chart 3":cluster{dbl, dbl, "Steering":dbl})
          }
          frame #6 {
            n194 = global read "G_ALL.vi" "CARDATA"() -> (w327:T6)
            n195 = global read "G_ALL.vi" "x origin"() -> (w326:dbl[])
            n196 = global read "G_ALL.vi" "y origin"() -> (w325:dbl[])
            n197 = call "Convert to Dynamic Data6"("Array"=w326) -> ("Dynamic Data Type"=w334:dynamicdata)  [unwired: 3 in]
            n198 = call "Convert to Dynamic Data7"("Array"=w325) -> ("Dynamic Data Type"=w333:dynamicdata)  [unwired: 3 in]
            n199 = Unbundle By Name(w327) -> ("x"=w331:dbl, "y"=w332:dbl)
            n200 = Merge Signals(w331, w334, w334) -> (w329:dynamicdata)
            n201 = Merge Signals(w332, w333, w333) -> (w328:dynamicdata)
            n202 = call "GRAPH"("Y Input"=w328, "X Input"=w329) -> ("XY Graph"=→"XY Graph 2":cluster{"Y":dbl[], "Y":dbl[]}[])  [unwired: 3 in, 6 out]
          }
        }
      }
      n203 = while {
        stop <- FALSE stop-if-true
        n204 = flat-sequence {
          frame #0 {
            # "Alert"
            n205 = Wait Until Next ms Multiple(millisecond multiple=u32 20 ("millisecond timer value")) -> ()  [unwired: 1 out]
          }
          frame #1 {
            n206 = global read "G_ALL.vi" "CARDATA"() -> (w195:T6)
            n207 = global read "G_ALL.vi" "beep"() -> (w196:T11)
            n208 = Unbundle By Name(w196) -> ("beep"=w193:bool, "frequency (Hz)"=w198:u32, "duration (msec)"=w197:u32)
            n209 = Unbundle By Name(w195) -> ("auto"=w194:bool)
            n210 = And(x=w194, y=w193) -> (x .and. y?=w192:bool)
            n211 = case shown="True" w192 {
              tunnel: w198 -> [_ w203]
              tunnel: w197 -> [_ w202]
              tunnel: w196 -> [_ w199]
              frame False {
              }
              frame True {
                w201 = FALSE ("use system alert? (T)")
                n212 = call <vilib>:"Beep.vi"("use system alert? (T)"=w201, "duration (msec)"=w202, "frequency (Hz)"=w203) -> ()  [unwired: 9 in]
                n213 = Bundle By Name(cluster=w199, "beep"=w201) -> (w200:T11)
                n214 = global write "G_ALL.vi" "beep"(w200) -> ()
              }
            }
          }
        }
      }
    }
  }
  n215 = flat-sequence {
    frame #0 {
      w335 = FALSE ("Make WPT")
      w339 = dbl[] [] ("x origin")
      w340 = FALSE ("Make WPT")
      n216 = local write "Path Num"(1 ("milliseconds to wait")) -> ()
      n217 = local write "lane keep"(FALSE ("lane update")) -> ()
      n218 = local write "mission auto"(TRUE ("mission auto")) -> ()
      n219 = local write "Laser lane"(w335) -> ()
      n220 = local write "Vision Lane"(w335) -> ()
      n221 = local write "Make WPT"(w340) -> ()
      n222 = local write "Load Path"(w340) -> ()
      n223 = global write "G_ALL.vi" "x origin"(w339) -> ()
      n224 = global write "G_ALL.vi" "y origin"(w339) -> ()
    }
    frame #1 {
      n225 = while {
        stop <- FALSE ("Loop 3") stop-if-true
        n226 = flat-sequence {
          frame #0 {
            n227 = Wait Until Next ms Multiple(millisecond multiple=u32 10 ("milliseconds to wait")) -> (millisecond timer value=w342:u32)
            n228 = feedback #3() -> (w344:u32)  [unwired: 1 in]
            n229 = feedback-in #3(w342) -> ()
            n230 = Subtract(x=w342, y=w344) -> (x-y=→"path":u32)
          }
          frame #1 {
            n231 = case shown="False" "Make WPT" {
              frame False {
                n232 = case shown="False" "Load Path" {
                  frame False {
                    n233 = flat-sequence {
                      frame #0 {
                        n234 = global read "G_LCM.vi" "car name"() -> (w348:string)
                        n235 = case shown="\"Avante\"" w348 {
                          selector: w348 -> [_ w351]
                          frame "Avante" {
                            n236 = flat-sequence {
                              frame #0 {
                                n237 = call "sick_ground filter.vi"() -> ()  [unwired: 12 in]
                              }
                              frame #1 {
                                n238 = disable-structure shown="Enabled" {
                                frame Disabled {
                                n239 = global read "G_ALL.vi" "mission num"() -> ()  [unwired: 1 out]
                                n240 = call "laneleftright41.vi"() -> ()  [unwired: 10 in, 2 out]
                                }
                                frame Enabled {
                                n241 = call "laneleftright5.vi"("update"="Vision Lane") -> ()  [unwired: 11 in]
                                }
                                }
                              }
                              frame #2 {
                                n242 = call "obsleftright.vi"("update"="Laser lane") -> ()  [unwired: 11 in]
                              }
                            }
                          }
                          frame Default {
                            n243 = flat-sequence {
                              tunnel: w351 -> [w352]
                              frame #0 {
                                n244 = case shown="\"Mobileye560\"" w352 {
                                frame Default {
                                n245 = call "mobileyelanepaser4.vi"("count hold"=u64 15, "thresh  c"=0.5, "thresh  b"=0.06 ("thresh 2"), "thresh r"=0.009 ("y")) -> ()  [unwired: 4 in, 4 out]
                                n246 = call "mobileyepaser.vi"() -> ()  [unwired: 11 in, 1 out]
                                }
                                frame "Mobileye560" {
                                n247 = global read "G_LCM.vi" "Mobileye_RAW_SNAP"() -> (w361:T14)
                                n248 = Unbundle By Name(w361) -> ("sys time"=w359:i64, "size"=w362:i32, "data"=w363:u8[])
                                n249 = feedback #4(i64 -1 ("sys time")) -> (w358:i64)
                                n250 = feedback-in #4(w359) -> ()
                                n251 = case shown="True" TRUE {
                                selector: TRUE -> [w364 _]
                                tunnel: w363 -> [_ w368]
                                tunnel: w362 -> [_ w365]
                                frame False {
                                n252 = global write "G_SEN.vi" "M_lane_update"(w364) -> ()
                                }
                                frame True {
                                n253 = Divide(x=w365, y=16) -> (x/y=w367:dbl)
                                n254 = for {
                                N: w367 -> [_]
                                tunnel: w368 -> [w389]
                                i -> [w388]
                                w381 = 4 ("length")
                                w379 = 8 ("index")
                                w387 = 16 ("y")
                                n255 = Multiply(x=w388, y=w387) -> (x*y=w386:i32)
                                n256 = Array Subset(array=w389, index=w386, length=w387) -> (w371:u8[])
                                n257 = Delete From Array(array=w371, length=w379, index=w379) -> (deleted portion=w372:u8[], array with subset deleted=w380:u8[])
                                n258 = Delete From Array(array=w380, length=w381, index=w381) -> (deleted portion=w385:u8[], array with subset deleted=w382:u8[])
                                n259 = Type Cast(type=u32 0, x=w382) -> (*(type *) &x=w373:u32)
                                n260 = Type Cast(type=u32 0, x=w385) -> (*(type *) &x=w374:u32)
                                n261 = Multiply(x=w374, y=1e-07) -> (x*y=w377:dbl)
                                n262 = To Time Stamp(1:w377) -> (0:w376:timestamp)
                                n263 = Bundle By Name(cluster=T12 {"identifier"=0, "timestamp"=timestamp(0 s since 1904-01-01), "payload"=[]} ("can cluster"), "identifier"=w373, "payload"=w372, "timestamp"=w376) -> (w370:T12)
                                n264 = call "mobileye_decoder_PC.vi"("can cluster"=w370, "name"="Mobileye560") -> ()  [unwired: 10 in]
                                }
                                }
                                }
                                n265 = Not Equal?(x=w359, y=w358) -> ()  [unwired: 1 out]
                                }
                                frame "Mobileye560S" {
                                n266 = global read "G_LCM.vi" "Mobileye_RAW_SNAP"() -> (w392:T14)
                                n267 = Unbundle By Name(w392) -> ("data"=w391:u8[])
                                n268 = Byte Array To String(unsigned byte array=w391) -> (string=w390:string)
                                n269 = while {
                                shift-right: [w395] -> _
                                shift-left: w390 -> [w397]
                                stop <- w396 stop-if-true
                                w401 = "S" ("regular expression")
                                n270 = Match Pattern(string=w397, regular expression="S") -> (after substring=w410:string)  [unwired: 1 in, 3 out]
                                n271 = Match Pattern(string=w410, regular expression=" ") -> (before substring=w408:string, after substring=w406:string)  [unwired: 1 in, 2 out]
                                n272 = Hexadecimal String To Number(string=w408) -> (number=w399:u32)  [unwired: 2 in, 1 out]
                                n273 = Match Pattern(string=w406, regular expression=w401) -> (before substring=w405:string, match substring=w402:string, after substring=w403:string)  [unwired: 1 in, 1 out]
                                n274 = Not Equal?(x=w402, y=w401) -> (x != y?=w396:bool)
                                n275 = Concatenate Strings(w402, w403) -> (w395:string)
                                n276 = for {
                                N: 8 -> [_]
                                tunnel: w405 -> [w419]
                                tunnel: [w415] -> w398 mode=indexing
                                i -> [w414]
                                n277 = Multiply(x=2, y=w414) -> (x*y=w417:i32)
                                n278 = String Subset(string=w419, offset (0)=w417, length (rest)=2 ("length (rest)")) -> (substring=w412:string)
                                n279 = Hexadecimal String To Number(string=w412, default (0uL)=u8 0) -> (number=w415:u8)  [unwired: 1 in, 1 out]
                                }
                                n280 = Get Date/Time In Seconds() -> (seconds since 1Jan1904=w404:timestamp)
                                n281 = Bundle By Name(cluster=T12 {"identifier"=0, "timestamp"=timestamp(0 s since 1904-01-01), "payload"=[]} ("can cluster"), "identifier"=w399, "payload"=w398, "timestamp"=w404) -> (w393:T12)
                                n282 = call "mobileye_decoder_PC.vi"("can cluster"=w393, "name"="Mobileye560") -> ()  [unwired: 10 in]
                                }
                                }
                                }
                              }
                              frame #1 {
                                n283 = global read "G_SEN.vi" "M_lane_update"() -> (w420:bool)
                                "Mobileye" <- w420
                                n284 = case shown="True" w420 {
                                frame False {
                                }
                                frame True {
                                n285 = global read "G_SEN.vi" "M_lane_center"() -> (w444:dbl[])
                                n286 = Index Array(array=w444, index=10) -> (element=w450:dbl)
                                n287 = Multiply(x=w450, y=10.0) -> (x*y=w461:dbl)
                                n288 = Round Toward -Infinity(1:w461) -> (0:w447:dbl)
                                n289 = global read "G_SEN.vi" "y_mobileye"() -> (w441:dbl[])
                                n290 = Max & Min(x=100.0, y=w447) -> (max(x,y)=w464:dbl)  [unwired: 1 out]
                                n291 = Array Subset(array=w441, index=0, length=w464) -> (w423:dbl[])
                                n292 = Index Array(array=w444, index #1=7 ("index"), index #2=6 ("index"), index #3=9 ("index"), index #4=5 ("index")) -> (element #1=w445:dbl, element #2=w458:dbl, element #3=w456:dbl, element #4=w463:dbl)
                                n293 = Square(x=w423) -> (x^2=w452:dbl[])
                                n294 = Array Subset(array=w423, index=1) -> (w435:dbl[])  [unwired: 1 in]
                                n295 = Array Size(array=w435) -> (size(s)=w432:i32)
                                n296 = Compound Arithmetic op=MULTIPLY(w445, w423, w452) -> (w455:dbl[])
                                n297 = Compound Arithmetic op=MULTIPLY(w452, w458) -> (w454:dbl[])
                                n298 = Compound Arithmetic op=MULTIPLY(w423, w456) -> (w453:dbl[])
                                n299 = Compound Arithmetic op=ADD(w455, w454, w453, w463) -> (w422:dbl[])
                                n300 = Array Subset(array=w423, index=0, length=w432) -> (w434:dbl[])
                                n301 = Build Array(w422, w423) -> (w442:dbl[][])
                                n302 = Array Subset(array=w422, index=1) -> (w436:dbl[])  [unwired: 1 in]
                                n303 = Subtract(x=w435, y=w434) -> (x-y=w430:dbl[])
                                n304 = Transpose 2D Array(2D array=w442) -> (transposed array=w443:dbl[][])
                                n305 = Array Size(array=w436) -> (size(s)=w439:i32)
                                n306 = global write "G_ALL.vi" "map_track lane"(w443) -> ()
                                n307 = Array Subset(array=w422, index=0, length=w439) -> (w437:dbl[])
                                n308 = Subtract(x=w436, y=w437) -> (x-y=w429:dbl[])
                                n309 = Square(x=w430) -> (x^2=w428:dbl[])
                                n310 = Square(x=w429) -> (x^2=w427:dbl[])
                                n311 = Add(x=w428, y=w427) -> (x+y=w426:dbl[])
                                n312 = Square Root(x=w426) -> (sqrt(x)=w425:dbl[])
                                n313 = Build Array (concatenate)(w425, 0.0) -> (w421:dbl[])
                                n314 = global write "G_ALL.vi" "dist lane"(w421) -> ()
                                }
                                }
                              }
                            }
                          }
                        }
                      }
                      frame #1 {
                        n315 = global read "G_ALL.vi" "x origin"() -> (w466:dbl[])
                        n316 = Empty Array?(array=w466) -> (empty?=w465:bool)
                        n317 = case shown="False" w465 {
                          frame False {
                            n318 = flat-sequence {
                              tunnel: [w473] -> w467
                              tunnel: w467 -> [w485]
                              frame #0 {
                                n319 = global read "G_ALL.vi" "mission num"() -> (w468:i32)
                                n320 = case shown="0, Default" w468 {
                                frame 0, Default {
                                }
                                frame 5 {
                                n321 = global read "G_LCM.vi" "VISION_FRONT_CAM"() -> (w470:T7)
                                n322 = Unbundle By Name(w470) -> ("sign"=w469:i32)
                                n323 = case shown="1..4" w469 {
                                selector: w469 -> [_ w471]
                                frame 0, Default {
                                }
                                frame 1..4 {
                                n324 = local write "Path Num"(w471) -> ()
                                }
                                }
                                }
                                }
                              }
                              frame #1 {
                                n325 = Multiply(x=0.1 ("y"), y="Global x shift") -> (x*y=w481:dbl)
                                n326 = Multiply(x="Global y shift", y=0.1) -> (x*y=w479:dbl)
                                n327 = call "tracking4.vi"("y"=w479, "x"=w481, "path num"="Path Num", "reset path"="reset path", "d"="d") -> ("mission"=w475:i32)  [unwired: 6 in]
                                n328 = Select(t=w475, s="mission auto", f="mission") -> (s? t:f=w473:i32)
                              }
                              frame #2 {
                                w486 = 0.0 ("x")
                                n329 = local write "mission"(w485) -> ()
                                n330 = global write "G_ALL.vi" "mission num"(w485) -> ()
                                n331 = local write "Global y shift"(w486) -> ()
                                n332 = local write "Global x shift"(w486) -> ()
                              }
                            }
                          }
                          frame True {
                            n333 = global write "G_ALL.vi" "STOP_LINE"(dbl[][] [] ("STOP_LINE")) -> ()
                          }
                        }
                      }
                      frame #2 {
                        n334 = global read "G_ALL.vi" "x origin"() -> (w493:dbl[])
                        n335 = Empty Array?(array=w493) -> (empty?=w492:bool)
                        n336 = Or(x="lane keep", y=w492) -> (x .or. y?=w489:bool)
                        n337 = disable-structure shown="Enabled" {
                          disable-tunnel: [w496 w498] -> w490
                          disable-tunnel: w489 -> [w495 w497]
                          disable-tunnel: [w494 w499] -> w488
                          frame Disabled {
                            n338 = call "path steer4.vi"("lane"=w495) -> ("curve vel limit"=w496:dbl, "handle"=w494:dbl)  [unwired: 9 in]
                          }
                          frame Enabled {
                            n339 = call "path steer7.vi"("lane"=w497) -> ("curve vel limit"=w498:dbl, "handle"=w499:dbl)  [unwired: 9 in]
                          }
                        }
                        n340 = global write "G_ALL.vi" "Steering"(w488) -> ()
                        n341 = global write "G_ALL.vi" "curve vel limit"(w490) -> ()
                      }
                    }
                  }
                  frame True {
                    n342 = flat-sequence {
                      tunnel: [w524] -> w508
                      tunnel: [w523] -> w505
                      tunnel: w508 -> [w552]
                      tunnel: [w552] -> w507
                      tunnel: w505 -> [w551]
                      tunnel: [w550] -> w504
                      tunnel: w507 -> [w574]
                      tunnel: [w574] -> w506
                      tunnel: w504 -> [w573]
                      tunnel: [w572] -> w503
                      tunnel: w506 -> [w596]
                      tunnel: [w596] -> w502
                      tunnel: w503 -> [w595]
                      tunnel: [w594] -> w500
                      tunnel: w502 -> [w617]
                      tunnel: [w617] -> w501
                      tunnel: w500 -> [w616]
                      tunnel: w501 -> [w641]
                      frame #0 {
                        w510 = FALSE ("X Scale.Loose Fit")
                        w509 = u8 0 ("X Scale.Scale Fit")
                        n343 = call "initvar.vi"() -> ()  [unwired: 12 in]
                        n344 = property on="XY Graph" class="XYGraph (strict)"("XScale.ScaleFit"=w509, "YScale.ScaleFit"=w509, "XScale.LooseFit"=w510, "YScale.LooseFit"=w510) -> ()  [unwired: 2 in, 2 out]
                      }
                      frame #1 {
                        n345 = Bundle("Minimum"=-5.0, "Minimum"=37.3, "Minimum"=10.0, "Minimum"=1.0, "Minimum"=-20.0) -> (w515:T15)  [unwired: 1 in]
                        n346 = Bundle("Minimum"=-22.6, "Minimum"=22.6, "Minimum"=10.0, "Minimum"=1.0, "Minimum"=-20.0) -> (w522:T15)  [unwired: 1 in]
                        n347 = property on="XY Graph" class="XYGraph (strict)"("XScale.Range"=w522) -> ()  [unwired: 2 in, 2 out]
                        n348 = property on="XY Graph" class="XYGraph (strict)"("YScale.Range"=w515) -> ()  [unwired: 2 in, 2 out]
                      }
                      frame #2 {
                        n349 = global read "G_ALL.vi" "file path"() -> (w525:path)
                        n350 = Build Path(base path=w525, name or relative path="wpt") -> (appended path=w526:path)
                        n351 = call "Read From Measurement File2"("Filename"=w526, "Reset"=TRUE) -> ("error out"=w529:errorcluster, "Filename Out"=w524:path, "Signals"=w531:dynamicdata)  [unwired: 4 in, 3 out]
                        n352 = Unbundle By Name(w529) -> ("status"=w528:bool)
                        n353 = case shown="False" w528 {
                          selector: w528 -> [_ w548]
                          tunnel: w531 -> [w533 _]
                          tunnel: [w532 w548] -> w523
                          frame False {
                            n354 = call "Convert from Dynamic Data2"("Dynamic Data Type"=w533) -> ("Array"=w535:dbl[][])  [unwired: 3 in]
                            n355 = Empty Array?(array=w535) -> (empty?=w534:bool)
                            n356 = case shown="False" w534 {
                              selector: w534 -> [w538 w546]
                              tunnel: w535 -> [w539 _]
                              tunnel: [w538 w546] -> w532
                              frame False {
                                n357 = global write "G_ALL.vi" "xym 1"(w539) -> ()
                                n358 = Index Array(array=w539, index (row) #1=6 ("index (row)"), index (row) #2=4 ("disabled index (col)"), index (row) #3=3 ("index (col)"), index (row) #4=7 ("index (row)")) -> (element #1=w536:dbl[], element #2=w545:dbl[], element #3=w544:dbl[], element #4=w540:dbl[])  [unwired: 4 in]
                                n359 = global write "G_ALL.vi" "v origin"(w536) -> ()
                                n360 = global write "G_ALL.vi" "x origin"(w545) -> ()
                                n361 = global write "G_ALL.vi" "y origin"(w544) -> ()
                                n362 = global write "G_ALL.vi" "mission"(w540) -> ()
                              }
                              frame True {
                                w547 = dbl[] [] ("x origin")
                                n363 = global write "G_ALL.vi" "x origin"(w547) -> ()
                                n364 = global write "G_ALL.vi" "y origin"(w547) -> ()
                              }
                            }
                          }
                          frame True {
                            w549 = dbl[] [] ("x origin")
                            n365 = global write "G_ALL.vi" "x origin"(w549) -> ()
                            n366 = global write "G_ALL.vi" "y origin"(w549) -> ()
                          }
                        }
                      }
                      frame #3 {
                        n367 = case shown="False" w551 {
                          selector: w551 -> [_ w571]
                          tunnel: [w553 w571] -> w550
                          frame False {
                            n368 = global read "G_ALL.vi" "file path"() -> (w561:path)
                            n369 = Build Path(base path=w561, name or relative path="wpt") -> (appended path=w560:path)
                            n370 = call "Read From Measurement File"("Filename"=w560, "Reset"=TRUE) -> ("error out"=w557:errorcluster, "Signals"=w555:dynamicdata)  [unwired: 4 in, 4 out]
                            n371 = Unbundle By Name(w557) -> ("status"=w558:bool)
                            n372 = case shown="False" w558 {
                              selector: w558 -> [_ w570]
                              tunnel: w555 -> [w564 _]
                              tunnel: [w563 _] -> w554
                              tunnel: [w562 w570] -> w553
                              frame False {
                                n373 = call "Convert from Dynamic Data"("Dynamic Data Type"=w564) -> ("Array"=w566:dbl[][])  [unwired: 3 in]
                                n374 = Empty Array?(array=w566) -> (empty?=w565:bool)
                                n375 = case shown="False" w565 {
                                selector: w565 -> [w567 w569]
                                tunnel: w566 -> [w568 _]
                                tunnel: [w568 _] -> w563
                                tunnel: [w567 w569] -> w562
                                frame False {
                                }
                                frame True {
                                }
                                }
                              }
                              frame True {
                              }
                            }
                            n376 = global write "G_ALL.vi" "xym 2"(w554) -> ()
                          }
                          frame True {
                          }
                        }
                      }
                      frame #4 {
                        n377 = case shown="True" w573 {
                          selector: w573 -> [_ w593]
                          tunnel: [w575 w593] -> w572
                          frame False {
                            n378 = global read "G_ALL.vi" "file path"() -> (w577:path)
                            n379 = Build Path(base path=w577, name or relative path="wpt") -> (appended path=w578:path)
                            n380 = call "Read From Measurement File3"("Filename"=w578, "Reset"=TRUE) -> ("error out"=w581:errorcluster, "Signals"=w583:dynamicdata)  [unwired: 4 in, 4 out]
                            n381 = Unbundle By Name(w581) -> ("status"=w580:bool)
                            n382 = case shown="True" w580 {
                              selector: w580 -> [_ w592]
                              tunnel: w583 -> [w586 _]
                              tunnel: [w585 _] -> w576
                              tunnel: [w584 w592] -> w575
                              frame False {
                                n383 = call "Convert from Dynamic Data3"("Dynamic Data Type"=w586) -> ("Array"=w588:dbl[][])  [unwired: 3 in]
                                n384 = Empty Array?(array=w588) -> (empty?=w587:bool)
                                n385 = case shown="False" w587 {
                                selector: w587 -> [w589 w591]
                                tunnel: w588 -> [w590 _]
                                tunnel: [w590 _] -> w585
                                tunnel: [w589 w591] -> w584
                                frame False {
                                }
                                frame True {
                                }
                                }
                              }
                              frame True {
                              }
                            }
                            n386 = global write "G_ALL.vi" "xym 3"(w576) -> ()
                          }
                          frame True {
                          }
                        }
                      }
                      frame #5 {
                        n387 = case shown="True" w595 {
                          selector: w595 -> [_ w615]
                          tunnel: [w597 w615] -> w594
                          frame False {
                            n388 = global read "G_ALL.vi" "file path"() -> (w605:path)
                            n389 = Build Path(base path=w605, name or relative path="wpt") -> (appended path=w604:path)
                            n390 = call "Read From Measurement File4"("Filename"=w604, "Reset"=TRUE) -> ("error out"=w601:errorcluster, "Signals"=w599:dynamicdata)  [unwired: 4 in, 4 out]
                            n391 = Unbundle By Name(w601) -> ("status"=w602:bool)
                            n392 = case shown="True" w602 {
                              selector: w602 -> [_ w614]
                              tunnel: w599 -> [w608 _]
                              tunnel: [w607 _] -> w598
                              tunnel: [w606 w614] -> w597
                              frame False {
                                n393 = call "Convert from Dynamic Data4"("Dynamic Data Type"=w608) -> ("Array"=w610:dbl[][])  [unwired: 3 in]
                                n394 = Empty Array?(array=w610) -> (empty?=w609:bool)
                                n395 = case shown="False" w609 {
                                selector: w609 -> [w611 w613]
                                tunnel: w610 -> [w612 _]
                                tunnel: [w612 _] -> w607
                                tunnel: [w611 w613] -> w606
                                frame False {
                                }
                                frame True {
                                }
                                }
                              }
                              frame True {
                              }
                            }
                            n396 = global write "G_ALL.vi" "xym 4"(w598) -> ()
                          }
                          frame True {
                          }
                        }
                      }
                      frame #6 {
                        n397 = case shown="False" w616 {
                          frame False {
                            n398 = global read "G_ALL.vi" "file path"() -> (w625:path)
                            n399 = Build Path(base path=w625, name or relative path="wpt") -> (appended path=w624:path)
                            n400 = call "Read From Measurement File5"("Filename"=w624, "Reset"=TRUE) -> ("error out"=w621:errorcluster, "Signals"=w619:dynamicdata)  [unwired: 4 in, 4 out]
                            n401 = Unbundle By Name(w621) -> ("status"=w622:bool)
                            n402 = case shown="False" w622 {
                              tunnel: w619 -> [w627 _]
                              tunnel: [w626 _] -> w618
                              frame False {
                                n403 = call "Convert from Dynamic Data5"("Dynamic Data Type"=w627) -> ("Array"=w629:dbl[][])  [unwired: 3 in]
                                n404 = Empty Array?(array=w629) -> (empty?=w628:bool)
                                n405 = case shown="False" w628 {
                                tunnel: w629 -> [w630 _]
                                tunnel: [w630 _] -> w626
                                frame False {
                                }
                                frame True {
                                }
                                }
                              }
                              frame True {
                              }
                            }
                            n406 = global write "G_ALL.vi" "xym 5"(w618) -> ()
                          }
                          frame True {
                          }
                        }
                      }
                      frame #7 {
                        n407 = Strip Path(path=w641) -> (name=w637:string)  [unwired: 1 out]
                        n408 = local write "Load Path"(FALSE ("Load WPT")) -> ()
                        n409 = local write "reset path"(TRUE ("reset path")) -> ()
                        n410 = Match Pattern(string=w637, regular expression="_") -> (after substring=w639:string)  [unwired: 1 in, 3 out]
                        n411 = Match Pattern(string=w639, regular expression=".lvm") -> (before substring=w636:string)  [unwired: 1 in, 3 out]
                        n412 = Scan From String(input string=w636, default 1=T13."KAIST" ("map name")) -> (error out=w635:errorcluster, output 1=w633:T13)  [unwired: 3 in, 2 out]
                        n413 = case shown="Error" w635 {
                          tunnel: [w646 w647] -> w634
                          tunnel: w633 -> [w646 _]
                          frame No Error {
                          }
                          frame Error {
                            n414 = global read "G_ALL.vi" "GPSDATA"() -> (w648:T16)
                            n415 = Unbundle By Name(w648) -> ("map_idx"=w647:i32)
                          }
                        }
                        n416 = call "mapconf.vi"("map name"=w634) -> ("y"=w643:cluster{dbl, dbl, "y":dbl, "y":dbl, dbl}, "x"=w644:cluster{dbl, dbl, "y":dbl, "y":dbl, dbl}, "new picture"=w645:picture)  [unwired: 8 in]
                        n417 = property on="XY Graph 2" class="XYGraph (strict)"("PlotImages.Back"=w645) -> ()  [unwired: 2 in, 2 out]
                        n418 = property on="XY Graph 2" class="XYGraph (strict)"("XScale.Range"=w644, "YScale.Range"=w643) -> ()  [unwired: 2 in, 2 out]
                      }
                    }
                  }
                }
              }
              frame True {
                n419 = flat-sequence {
                  tunnel: [w652] -> w649
                  tunnel: w649 -> [w720]
                  frame #0 {
                    w650 = 0.0
                    n420 = global write "G_ALL.vi" "VS_des"(w650) -> ()
                    n421 = global write "G_ALL.vi" "Steering"(w650) -> ()
                  }
                  frame #1 {
                    n422 = local read "Make WPT"() -> (w651:bool)
                    n423 = Initialize Array(0.0 ("element"), 7 ("dimension size"), 1 ("dimension size")) -> (w653:dbl[][])
                    n424 = while {
                      shift-right: [w657] -> w652
                      shift-left: w653 -> [w659]
                      shift-right: [FALSE] -> _
                      shift-left: w651 -> [w660]
                      stop <- w662 stop-if-true
                      n425 = flat-sequence {
                        tunnel: [w674] -> w658
                        frame #0 {
                          n426 = global read "G_ALL.vi" "GPSDATA"() -> (w669:T16)
                          n427 = global read "G_ALL.vi" "CARDATA"() -> (w668:T6)
                          n428 = Unbundle By Name(w669) -> ("lat"=w673:dbl, "lon"=w672:dbl, "hgt"=w671:dbl, "map_idx"=w667:i32)
                          n429 = Unbundle By Name(w668) -> ("y"=w665:dbl, "x"=w664:dbl, "VS_can"=w666:dbl)
                          n430 = To Double Precision Float(number=w667) -> (double precision float=w670:dbl)
                          n431 = Build Array(w673, w672, w671, w665, w664, w671, w666, w670) -> (w674:dbl[])
                        }
                      }
                      n432 = local read "Make WPT"() -> (w663:bool)
                      n433 = Not(x=w663) -> (.not. x?=w662:bool)
                      n434 = case shown="False" w660 {
                        tunnel: w659 -> [w689 w706]
                        tunnel: w658 -> [w688 w704]
                        tunnel: [w687 w703] -> w657
                        frame False {
                          n435 = Array Size(array=w689) -> (size(s)=w697:i32[])
                          n436 = Index Array(array=w688, index #1=3 ("index"), index #2=4 ("index")) -> (element #1=w683:dbl, element #2=w681:dbl)
                          n437 = Index Array(array=w697, index=1) -> (element=w686:i32)
                          n438 = Decrement(x=w686) -> (x-1=w685:i32)
                          n439 = Index Array(array=w689, index (col)=w685) -> (element=w693:dbl[])  [unwired: 1 in]
                          n440 = Index Array(array=w693, index #1=3 ("index"), index #2=4 ("index")) -> (element #1=w684:dbl, element #2=w682:dbl)
                          n441 = Subtract(x=w684, y=w683) -> (x-y=w680:dbl)
                          n442 = Subtract(x=w682, y=w681) -> (x-y=w679:dbl)
                          n443 = Square(x=w680) -> (x^2=w678:dbl)
                          n444 = Square(x=w679) -> (x^2=w677:dbl)
                          n445 = Add(x=w678, y=w677) -> (x+y=w676:dbl)
                          n446 = Greater Or Equal?(x=w676, y=0.25) -> (x >= y?=w690:bool)
                          n447 = case shown="True" w690 {
                            tunnel: w689 -> [w698 w702]
                            tunnel: w686 -> [_ w699]
                            tunnel: w688 -> [_ w701]
                            tunnel: [w698 w700] -> w687
                            frame False {
                            }
                            frame True {
                              n448 = Insert Into Array(array=w702, index (col)=w699, new element=w701) -> (w700:dbl[][])  [unwired: 1 in]
                            }
                          }
                        }
                        frame True {
                          n449 = Replace Array Subset(array=w706, new element=w704, index (col)=0 ("disabled index (col)")) -> (w703:dbl[][])  [unwired: 1 in]
                        }
                      }
                    }
                  }
                  frame #2 {
                    n450 = call "Convert to Dynamic Data"("2D Array"=w720) -> ("Dynamic Data Type"=w721:dynamicdata)  [unwired: 3 in]
                    n451 = global read "G_ALL.vi" "GPSDATA"() -> (w710:T16)
                    n452 = Unbundle By Name(w710) -> ("map_idx"=w708:i32)
                    n453 = Get Date/Time In Seconds() -> (seconds since 1Jan1904=w718:timestamp)
                    n454 = Format Date/Time String(time format string (%c)="%2y%2m%2d%2H%2M", seconds (now)=w718) -> (date/time string=w716:string)  [unwired: 1 in]
                    n455 = Format Into String(w708) -> (resulting string=w707:string)  [unwired: 3 in, 1 out]
                    n456 = global read "G_ALL.vi" "file path"() -> (w709:path)
                    n457 = Build Path(base path=w709, name or relative path="wpt") -> (appended path=w713:path)
                    n458 = Concatenate Strings(w716, "_" ("string"), w707, ".lvm" ("string")) -> (w712:string)
                    n459 = Build Path(base path=w713, name or relative path=w712) -> (appended path=w711:path)
                    n460 = call "save wpt"("Signals"=w721, "Reset"=TRUE, "Filename"=w711) -> ()  [unwired: 14 in, 3 out]
                  }
                }
              }
            }
          }
        }
      }
    }
  }
  n461 = flat-sequence {
    frame #0 {
      # "Sensor paser"
    }
    frame #1 {
      w724 = dbl[][] [] ("M_lane_left")
      w725 = dbl[] [] ("M_lane_left")
      n462 = global write "G_SEN.vi" "vision y shift"(0.0 ("vision y shift")) -> ()
      n463 = local write "Log"(FALSE ("obs")) -> ()
      n464 = global write "G_SEN.vi" "sensor_obs"(w724) -> ()
      n465 = global write "G_SEN.vi" "sensor_lane"(w724) -> ()
      n466 = global write "G_SEN.vi" "M_lane_left"(w725) -> ()
      n467 = global write "G_SEN.vi" "M_lane_right"(w725) -> ()
      n468 = global write "G_SEN.vi" "M_lane_center"(w725) -> ()
    }
    frame #2 {
      n469 = while {
        stop <- FALSE ("Loop 4") stop-if-true
        n470 = flat-sequence {
          frame #0 {
            n471 = disable-structure shown="Enabled" {
              disable-tunnel: [w731 w733] -> w728
              frame Enabled {
                n472 = Wait Until Next ms Multiple(millisecond multiple=u32 10 ("milliseconds to wait")) -> (millisecond timer value=w731:u32)
              }
              frame Disabled {
                n473 = Tick Count (ms)() -> (millisecond timer value=w733:u32)
              }
            }
            n474 = feedback #5() -> (w730:u32)  [unwired: 1 in]
            n475 = feedback-in #5(w728) -> ()
            n476 = Subtract(x=w728, y=w730) -> (x-y=→"sensor":u32)
          }
          frame #1 {
            n477 = disable-structure shown="Disabled" {
              frame Disabled {
                n478 = flat-sequence {
                  frame #0 {
                    w735 = 0.0 ("roll")
                    n479 = call "velosterpaser384.vi"("roll"=w735, "pitch"=w735, "heading"=w735, "dX"=w735, "dY"=w735, "dZ"=w735, "Velodyne"=T17."Velodyne 16") -> ()  [unwired: 12 in, 1 out]
                  }
                  frame #1 {
                    w736 = 0.0 ("roll")
                    n480 = call "velosterpaser384.vi"("roll"=w736, "pitch"=w736, "heading"=w736, "dX"=w736, "dY"=w736, "dZ"=w736, "Velodyne"=T17."Velodyne 64") -> ()  [unwired: 12 in, 1 out]
                  }
                  frame #2 {
                    w743 = TRUE ("Sensor [F12]")
                    n481 = call "Ibeopaser.vi"("theta"=-2.5, "Hide Transparent"=w743, "Sensor [F12]"=w743) -> ("x_sensor"=w739:cluster{"idx":i32, "x":dbl, "y":dbl, "h":dbl}, "etc"=w741:dbl[][], "lane"=w740:dbl[][], "obs"=w738:dbl[][], "update"=w742:bool)  [unwired: 4 in]
                    n482 = case shown="True" w742 {
                      tunnel: w738 -> [_ w750]
                      tunnel: w739 -> [_ w745]
                      tunnel: w740 -> [_ w747]
                      tunnel: w741 -> [_ w748]
                      frame False {
                      }
                      frame True {
                        n483 = disable-structure shown="Enabled" {
                          disable-tunnel: w750 -> [w755 w757]
                          disable-tunnel: [w754 w757] -> w749
                          disable-tunnel: w748 -> [w753 _]
                          disable-tunnel: w747 -> [w752 w756]
                          disable-tunnel: [w751 w756] -> w746
                          frame Disabled {
                            n484 = call "test3.vi"("sensor_all"=w753, "sensor_lane"=w752, "sensor_obs"=w755) -> ("lane"=w751:dbl[][], "obs"=w754:dbl[][])  [unwired: 6 in, 1 out]
                          }
                          frame Enabled {
                          }
                        }
                        n485 = global write "G_ALL.vi" "x_ibeo"(w745) -> ()
                        n486 = global write "G_SEN.vi" "sensor_obs"(w749) -> ()
                        n487 = global write "G_SEN.vi" "sensor_lane"(w746) -> ()
                      }
                    }
                  }
                }
              }
              frame Enabled {
              }
              frame Disabled {
                n488 = call "velosterpaserraw.vi"() -> ()  [unwired: 20 in]
              }
            }
          }
          frame #2 {
            n489 = disable-structure shown="Enabled" {
              frame Disabled {
                n490 = global read "G_ALL.vi" "x_ibeo"() -> (w759:cluster{"idx":i32, "x":dbl, "y":dbl, "h":dbl})
                n491 = disable-structure shown="Disabled" {
                  disable-tunnel: [w786 w820] -> w760
                  disable-tunnel: w759 -> [w772 w819]
                  disable-tunnel: [w771 w819] -> w758
                  frame Disabled {
                    n492 = global read "G_ALL.vi" "CARDATA"() -> (w773:T6)
                    n493 = global read "G_SEN.vi" "Lane_R_M"() -> (w795:dbl[])
                    n494 = global read "G_SEN.vi" "Lane_L_M"() -> (w792:dbl[])
                    n495 = Unbundle By Name(w773) -> ("x"=w770:dbl, "y"=w769:dbl, "heading"=w768:dbl)
                    n496 = Index Array(array=w795, index=0) -> (element=w797:dbl)
                    n497 = Index Array(array=w792, index=0) -> (element=w790:dbl)
                    n498 = Bundle By Name(cluster=w772, "x"=w770, "y"=w769, "h"=w768) -> (w771:cluster{"idx":i32, "x":dbl, "y":dbl, "h":dbl})
                    n499 = Greater?(x=w797, y=0.65) -> (0:w796:bool)
                    n500 = Greater?(x=w790, y=0.65) -> (0:w791:bool)
                    n501 = case shown="True" w796 {
                      tunnel: w795 -> [_ w810]
                      tunnel: [_ w811] -> w781
                      tunnel: [_ w809] -> w780
                      frame False {
                      }
                      frame True {
                        n502 = global read "G_SEN.vi" "y_mobileye"() -> (w809:dbl[])
                        n503 = Index Array(array=w810, index #1=1 ("index")) -> (element #1=w816:dbl, element #2=w815:dbl, element #3=w812:dbl)  [unwired: 2 in]
                        n504 = Square(x=w809) -> (x^2=w817:dbl[])
                        n505 = Multiply(x=w815, y=w809) -> (x*y=w813:dbl[])
                        n506 = Multiply(x=w816, y=w817) -> (x*y=w814:dbl[])
                        n507 = Compound Arithmetic op=ADD(w814, w813, w812) -> (w811:dbl[])
                      }
                    }
                    n508 = case shown="True" w791 {
                      tunnel: w792 -> [_ w800]
                      tunnel: [_ w801] -> w779
                      tunnel: [_ w799] -> w778
                      frame False {
                      }
                      frame True {
                        n509 = global read "G_SEN.vi" "y_mobileye"() -> (w799:dbl[])
                        n510 = Index Array(array=w800, index #1=1 ("index")) -> (element #1=w806:dbl, element #2=w805:dbl, element #3=w802:dbl)  [unwired: 2 in]
                        n511 = Square(x=w799) -> (x^2=w807:dbl[])
                        n512 = Multiply(x=w805, y=w799) -> (x*y=w803:dbl[])
                        n513 = Multiply(x=w806, y=w807) -> (x*y=w804:dbl[])
                        n514 = Compound Arithmetic op=ADD(w804, w803, w802) -> (w801:dbl[])
                      }
                    }
                    n515 = Build Array(w781, w780) -> (w785:dbl[][])
                    n516 = Build Array(w779, w778) -> (w783:dbl[][])
                    n517 = Array Subset(array=w785, index (col)=0 ("index"), length (col)=5 ("length")) -> (w784:dbl[][])  [unwired: 2 in]
                    n518 = Array Subset(array=w783, index (col)=0 ("index"), length (col)=5 ("length")) -> (w782:dbl[][])  [unwired: 2 in]
                    n519 = Transpose 2D Array(2D array=w784) -> (transposed array=w788:dbl[][])
                    n520 = Transpose 2D Array(2D array=w782) -> (transposed array=w787:dbl[][])
                    n521 = Build Array (concatenate)(w788, w787) -> (w786:dbl[][])
                  }
                  frame Enabled {
                    n522 = global read "G_SEN.vi" "sensor_obs"() -> (w820:dbl[][])
                  }
                }
                n523 = global read "G_SEN.vi" "sensor_obs_log"() -> (w764:dbl[][])
                n524 = call "sensor_log2.vi"("xmax"=999999999.0, "FF"=1.0 ("t"), "xmin"=-99999999.0, "x_sensor"=w758, "ymin"=-99999999.0, "ymax"=99999999.0, "sensor_log in"=w764, "sensor_obs"=w760) -> ("sensor_log out"=w763:dbl[][])  [unwired: 3 in]
                n525 = global write "G_SEN.vi" "sensor_obs_log"(w763) -> ()
              }
              frame Enabled {
                n526 = case shown="True" "Log" {
                  frame False {
                    n527 = disable-structure shown="Enabled" {
                      frame Enabled {
                        n528 = global write "G_SEN.vi" "sensor_obs_log"(dbl[][] [] ("sensor_obs_log")) -> ()
                      }
                      frame Disabled {
                      }
                    }
                  }
                  frame True {
                    n529 = global read "G_ALL.vi" "mission num"() -> (w826:i32)
                    n530 = global read "G_ALL.vi" "CARDATA"() -> (w827:T6)
                    n531 = case shown="2, 4, 6" w826 {
                      tunnel: [_ TRUE] -> w824
                      frame 0, Default {
                      }
                      frame 2, 4, 6 {
                      }
                    }
                    n532 = Unbundle By Name(w827) -> ("VS_can"=w828:dbl)
                    n533 = Not Equal To 0?(x=w828) -> (x != 0?=w825:bool)
                    n534 = And(x=w825, y=w824) -> (x .and. y?=w823:bool)
                    n535 = case shown="True" w823 {
                      frame False {
                      }
                      frame True {
                        n536 = disable-structure shown="Enabled" {
                          disable-tunnel: [w850 w852 w854] -> w834
                          disable-tunnel: [w849 w851 w853] -> w830
                          frame Disabled {
                            n537 = global read "G_SEN.vi" "sensor_obs"() -> (w850:dbl[][])
                            n538 = global read "G_ALL.vi" "x_ibeo"() -> (w849:cluster{"idx":i32, "x":dbl, "y":dbl, "h":dbl})
                          }
                          frame Enabled {
                            n539 = global read "G_ALL.vi" "x_sick_front"() -> (w851:cluster{"idx":i32, "x":dbl, "y":dbl, "h":dbl})
                            n540 = global read "G_SEN.vi" "SICK_laser"() -> (w852:dbl[][])
                          }
                          frame Disabled {
                            n541 = global read "G_LCM.vi" "VISION_LANE_PT"() -> (w859:T18)
                            n542 = Unbundle By Name(w859) -> ("x"=w858:dbl[], "y"=w857:dbl[], "point_flag"=w856:i32[])
                            n543 = Build Array(w858, w857, w856) -> (w855:dbl[][])
                            n544 = global read "G_ALL.vi" "x_AVM"() -> (w853:cluster{"idx":i32, "x":dbl, "y":dbl, "h":dbl})
                            n545 = Transpose 2D Array(2D array=w855) -> (transposed array=w854:dbl[][])
                          }
                        }
                        n546 = disable-structure shown="Enabled" {
                          disable-tunnel: [15.0 ("ymax") 5000.0 ("ymax")] -> w838
                          disable-tunnel: [-5.0 ("ymin") -5000.0 ("ymin")] -> w837
                          disable-tunnel: [5.0 ("xmax") 5000.0 ("xmax")] -> w836
                          disable-tunnel: [-3.0 ("xmin") -5000.0 ("xmin")] -> w835
                          disable-tunnel: [0.99 ("t") 1.0 ("FF")] -> w831
                          frame Disabled {
                          }
                          frame Enabled {
                          }
                        }
                        n547 = global read "G_SEN.vi" "sensor_obs_log"() -> (w833:dbl[][])
                        n548 = call "sensor_log2.vi"("xmax"=w836, "FF"=w831, "xmin"=w835, "x_sensor"=w830, "ymin"=w837, "ymax"=w838, "sensor_log in"=w833, "sensor_obs"=w834) -> ("sensor_log out"=w832:dbl[][])  [unwired: 3 in]
                        n549 = global write "G_SEN.vi" "sensor_obs_log"(w832) -> ()
                      }
                    }
                  }
                }
              }
            }
          }
        }
      }
    }
  }
